vi "Fluke5000.vi"(4 "error in":T13, 7 "Command":T14) -> (0 "error out":T13, 3 "Response":T11)   [LabVIEW 2018]
uses:
  MOKO_LabViewLibrary/MokoLowLevel/MokoLowLovelControl/MLLC_Command.ctl
  MOKO_LabViewLibrary/MokoLowLevel/MokoLowLovelControl/MLLC_Error.ctl
  MOKO_LabViewLibrary/MokoLowLevel/MokoLowLovelControl/MLLC_Mode.ctl
  MOKO_LabViewLibrary/MokoLowLevel/MokoLowLovelControl/MLLC_Response.ctl
  MOKO_LabViewLibrary/MokoLowLevel/MokoLowLovelControl/MLLC_DriverName.ctl
  MOKO_LabViewLibrary/MokoLowLevel/MokoLowLovelControl/MLLC_Request.ctl
  MOKO_LabViewLibrary/MokoLowLevel/MokoLowLovelControl/MLLC_ErrorCode.ctl
  MOKO_LabViewLibrary/MokoLowLevel/MokoLowLovelControl/MLLC_ResponseInit.ctl
  MOKO_LabViewLibrary/MokoLowLevel/MokoLowLovelControl/MLLC_ConnectCluster.ctl
  MOKO_LabViewLibrary/MokoLowLevel/MokoLowLovelControl/MLLC_InterfaceType.ctl
  MOKO_LabViewLibrary/MokoLowLevel/MokoLowLovelControl/MLLC_OpenedSession.ctl
  MOKO_LabViewLibrary/MokoLowLevel/MokoLowLovelControl/MLLC_InterfaceSettings.ctl
  MOKO_LabViewLibrary/MokoLowLevel/MokoLowLovelControl/MLLC_InterfaceKind.ctl
  data/Models.ctl
panel:
  in  "Settings":T6={"Permanent data"={"Connect"={"InterfaceType"=enum."VISA", "OpenedSession"="COM1", "InterfaceSettings"={"Interface"=enum."GPIB", "EOS 4 read"=enum."LF (\\n)", "EOS 4 write"=enum."LF (\\n)", "TMO, ms"=5000, "Sett"=variant(cluster{"Baud Rate":u32, "Data Bits":u16, "Parity":u16, "Stop Bits":u16, "Flow Control":u16, "Eho":bool} {"Baud Rate"=75, "Data Bits"=0, "Parity"=0, "Stop Bits"=0, "Flow Control"=0, "Eho"=FALSE})}}, "Conn"=2, "Model"=0.0, "Channel"="CH1", "Impedance"="Z1M", "SwitchOFF"=TRUE, "Out"="NORMAL", "OutSignalAuto"=TRUE, "PQ"=FALSE}, "Saved Data"=variant} {"Permanent data"."Conn" items=["2-Wire", "4-Wire", "NONE"]}
  in  "Response Init Array":T7[](array[typedef])=["5500", "5502", "5520", "5522", "5700", "5720", "5730"]
  in  "Error Code":T8=5470
  in  "Request":T9="*idn?"
  in  "Driver Name":T10="Fluke5000"
  in  "Mode":T12=enum."Check"
  # "F5000"
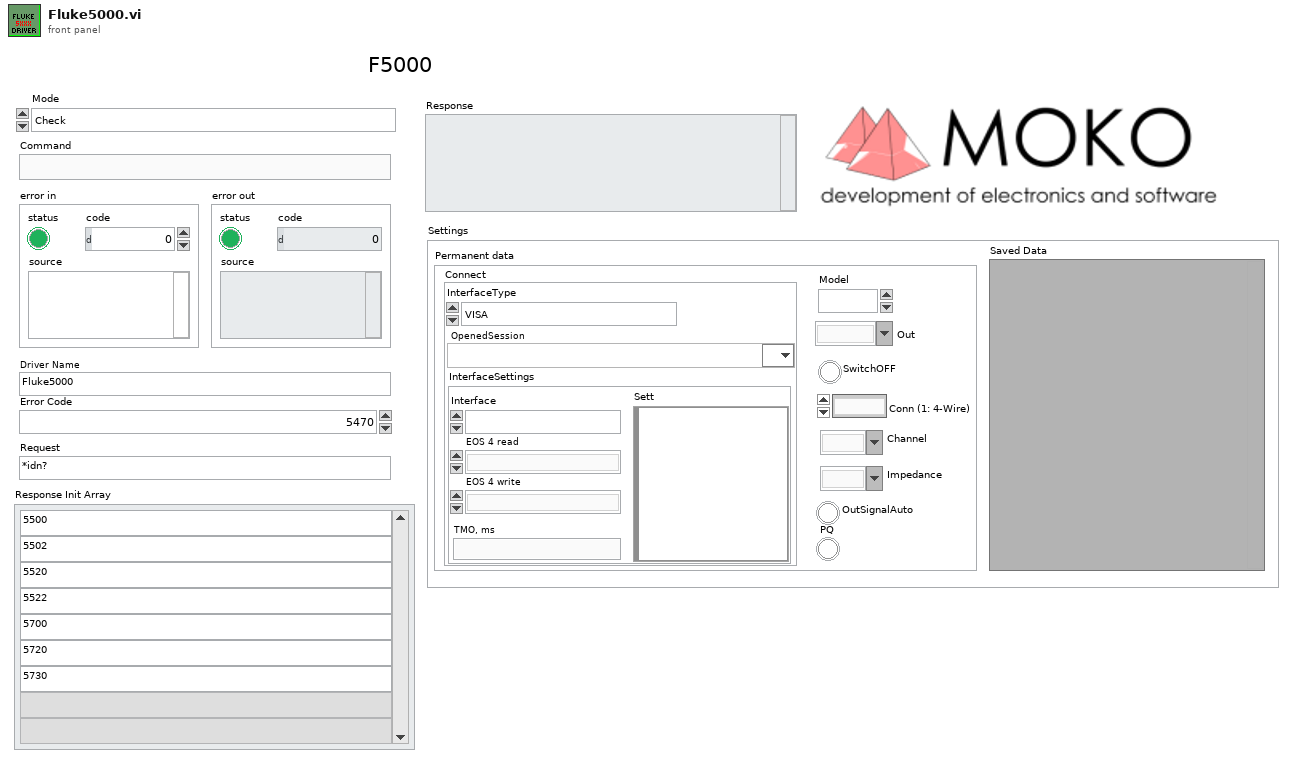
[diagram p1: front panel]
types:
  T1 = typedef "MLLC_ConnectCluster.ctl" = cluster{"InterfaceType":T2, "OpenedSession":T3, "InterfaceSettings":T4}
  T2 = typedef "MLLC_InterfaceType.ctl" = enum16{"VISA", "Prologix USB-GPIB"}
  T3 = typedef "MLLC_OpenedSession.ctl" = refnum<visa-resource-name>
  T4 = typedef "MLLC_InterfaceSettings.ctl" = cluster{"Interface":T5, "EOS 4 read":enum16{"Default (=EOS 4 write)", "CR (\\r)", "LF (\\n)", "None"}, "EOS 4 write":enum16{"CR+LF (\\r\\n)", "CR (\\r)", "LF (\\n)", "None"}, "TMO, ms":i32, "Sett":variant}
  T5 = typedef "MLLC_InterfaceKind.ctl" = enum16{"RS232", "GPIB", "USB", "Ethernet", "another"}
  T6 = cluster{"Permanent data":cluster{"Connect":T1, "Conn":u16, "Model":dbl, "Channel":string, "Impedance":string, "SwitchOFF":bool, "Out":string, "OutSignalAuto":bool, "PQ":bool}, "Saved Data":variant}
  T7 = typedef "MLLC_ResponseInit.ctl" = string
  T8 = typedef "MLLC_ErrorCode.ctl" = u32
  T9 = typedef "MLLC_Request.ctl" = string
  T10 = typedef "MLLC_DriverName.ctl" = string
  T11 = typedef "MLLC_Response.ctl" = string
  T12 = typedef "MLLC_Mode.ctl" = enum16{"get", "set", "close", "Init", "Check"}
  T13 = typedef "MLLC_Error.ctl" = errorcluster
  T14 = typedef "MLLC_Command.ctl" = string
  T15 = enum16{"CR+LF (\\r\\n)", "CR (\\r)", "LF (\\n)", "None"}
  T16 = enum16{"Default (=EOS 4 write)", "CR (\\r)", "LF (\\n)", "None"}
  T17 = cluster{"Connect":T1, "Conn":u16, "Model":dbl, "Channel":string, "Impedance":string, "SwitchOFF":bool, "Out":string, "OutSignalAuto":bool, "PQ":bool}
  T18 = typedef "Models.ctl" = enum16{"5500", "5520", "5700", "5720", "5502", "5522", "5730"}
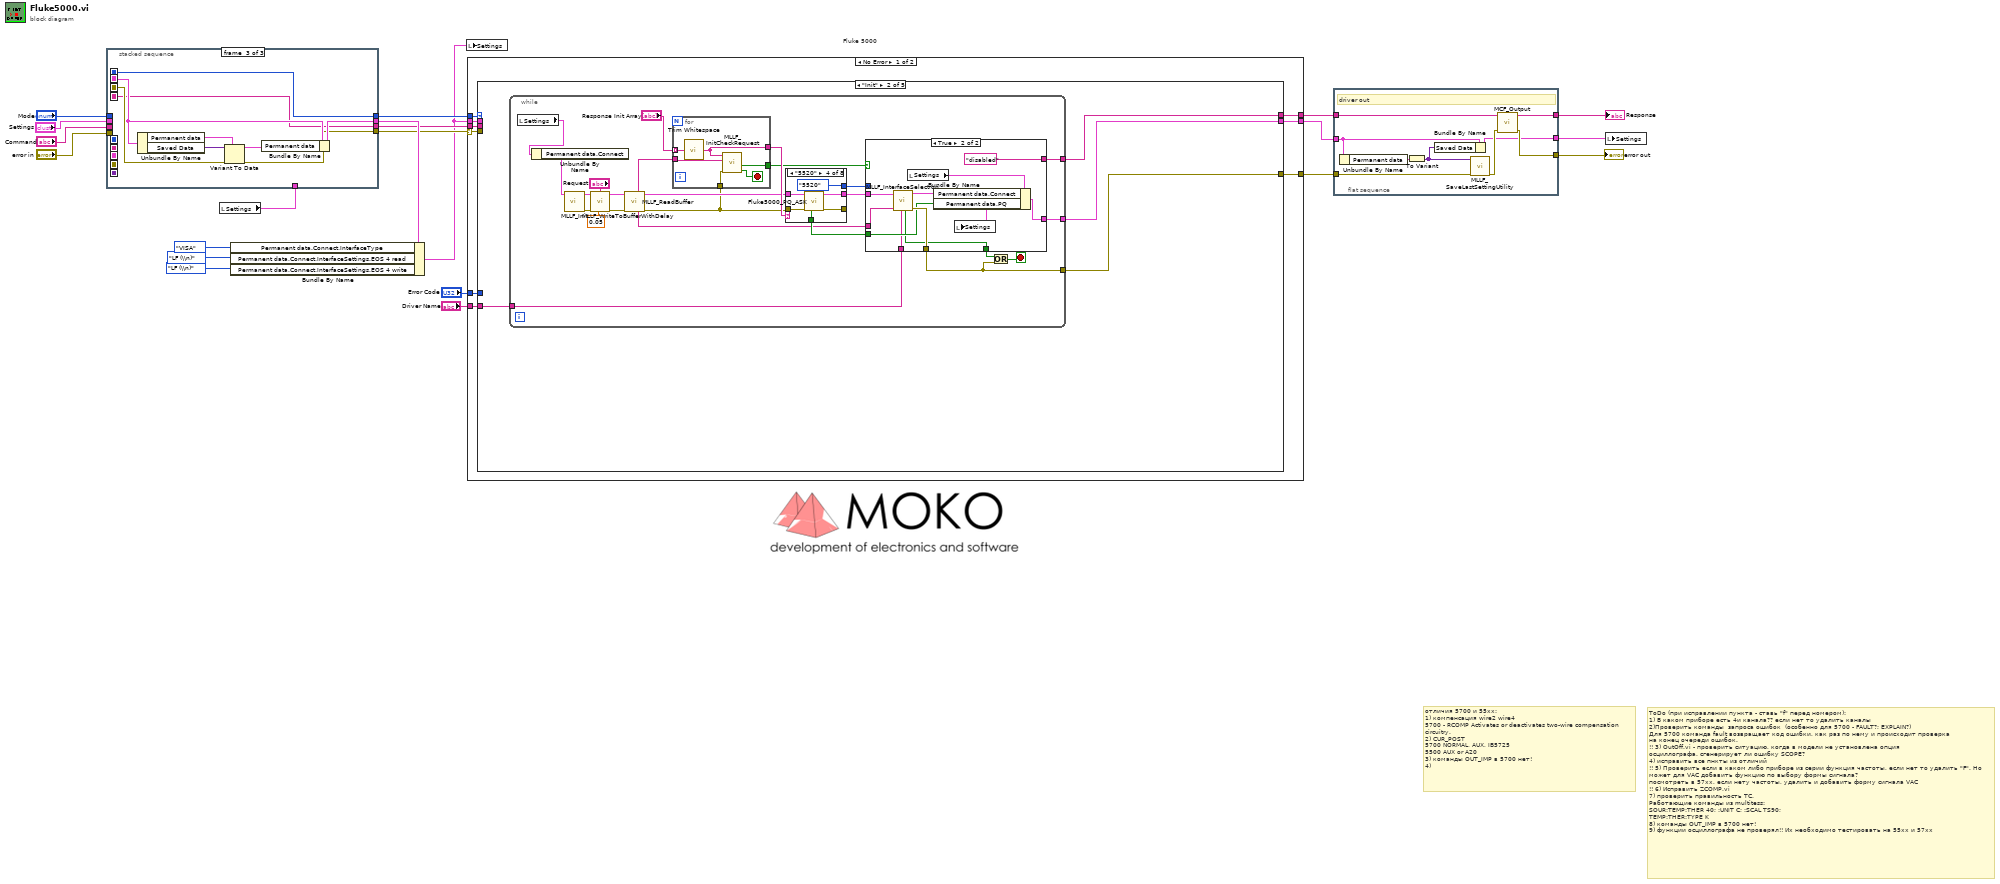
[diagram p0: block diagram]
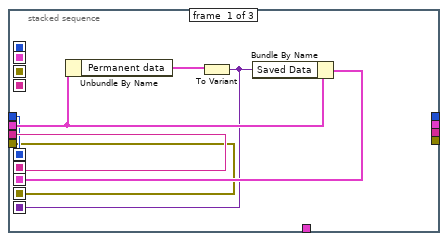
[diagram p2: hidden frame]
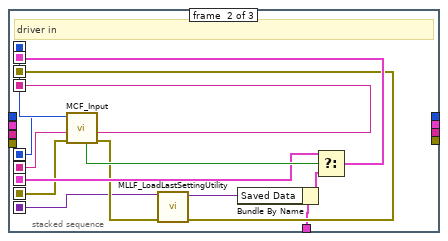
[diagram p3: hidden frame]
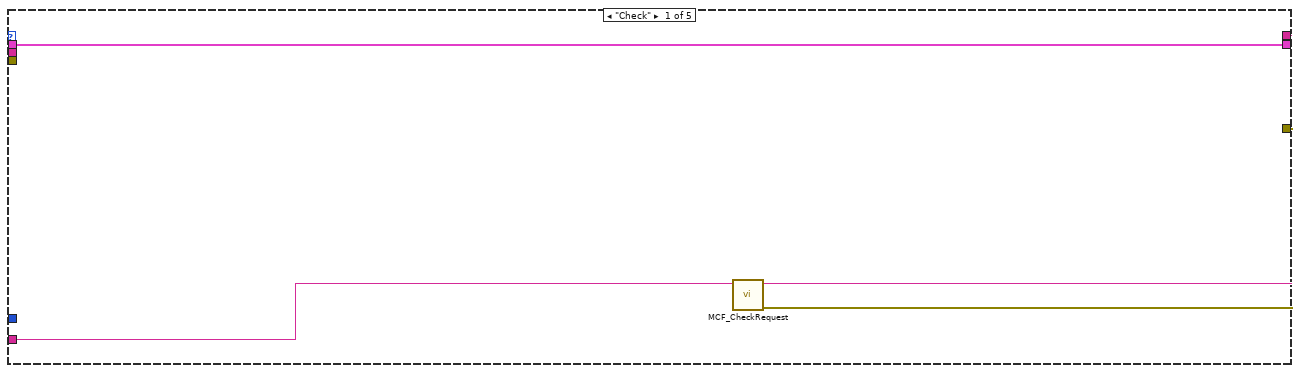
[diagram p4: hidden frame]
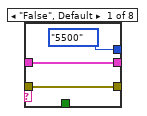
[diagram p5: hidden frame]
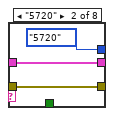
[diagram p6: hidden frame]
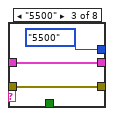
[diagram p7: hidden frame]
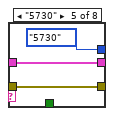
[diagram p8: hidden frame]
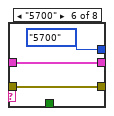
[diagram p9: hidden frame]
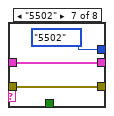
[diagram p10: hidden frame]
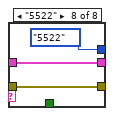
[diagram p11: hidden frame]
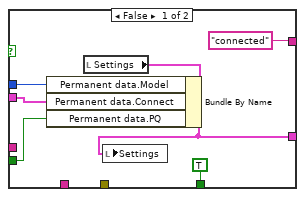
[diagram p12: hidden frame]
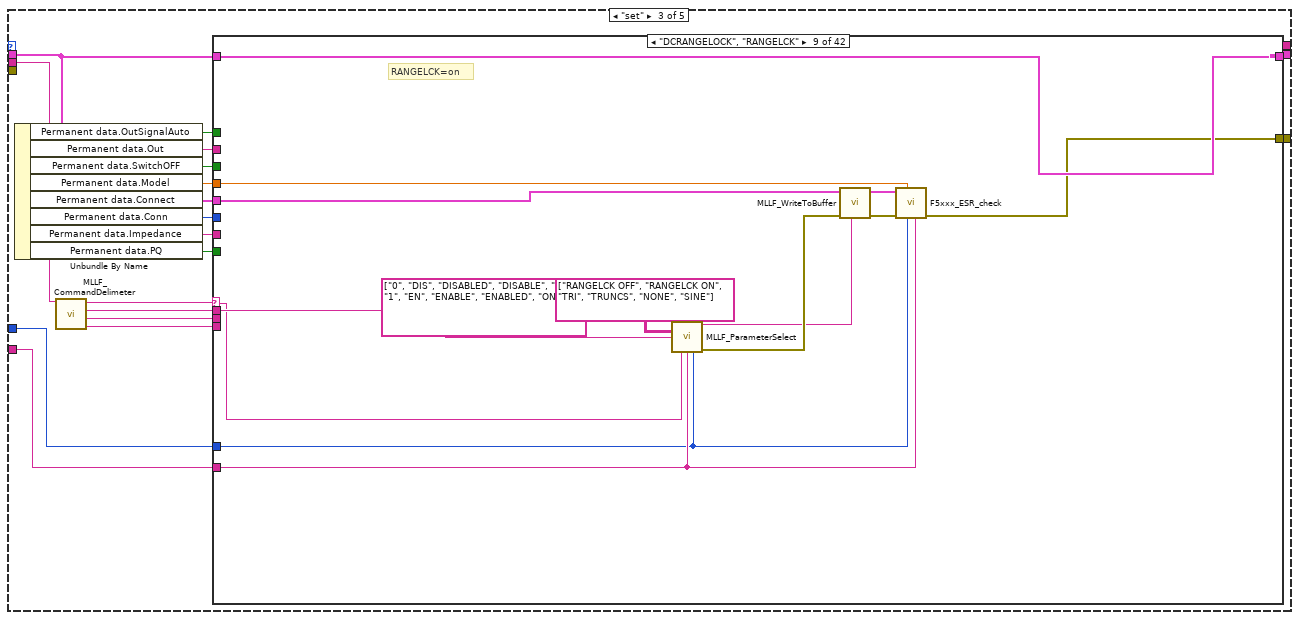
[diagram p13: hidden frame]
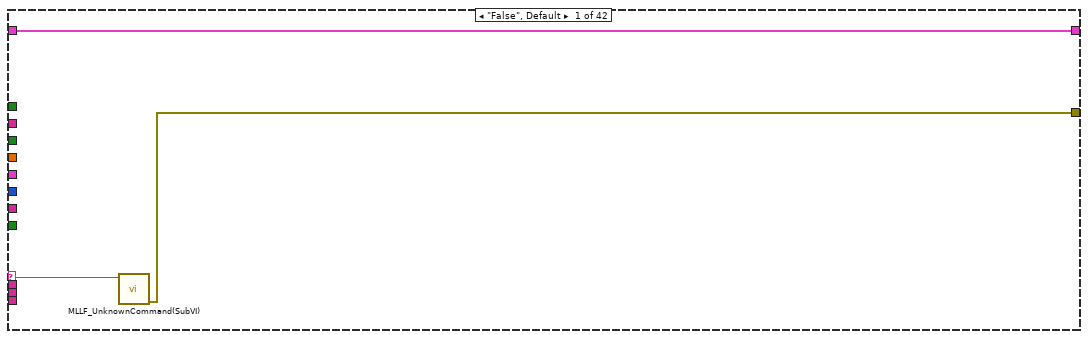
[diagram p14: hidden frame]
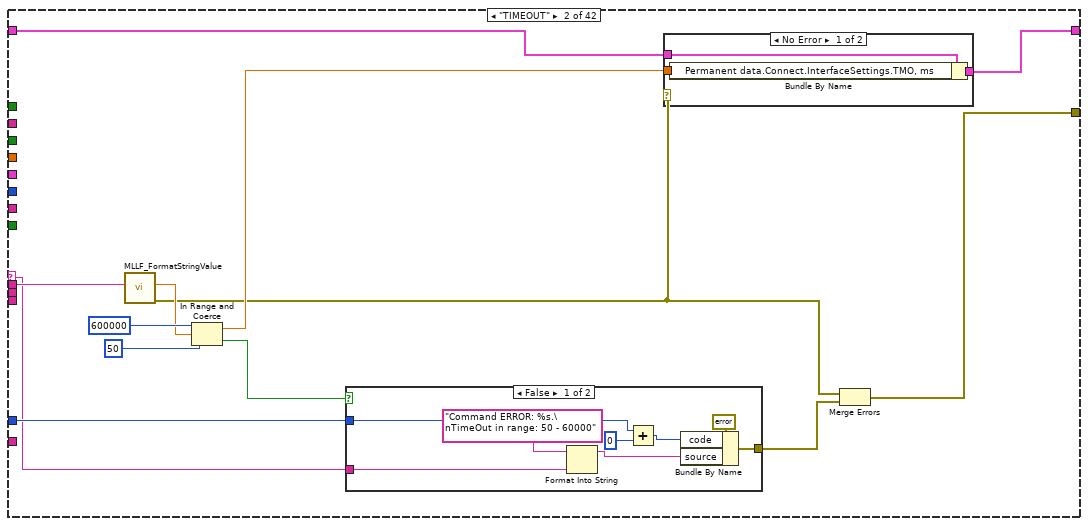
[diagram p15: hidden frame]
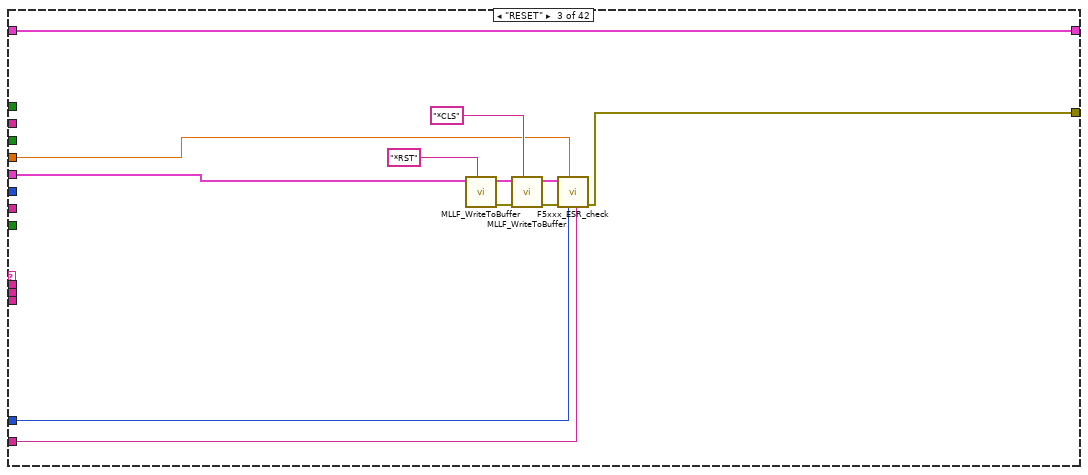
[diagram p18: hidden frame]
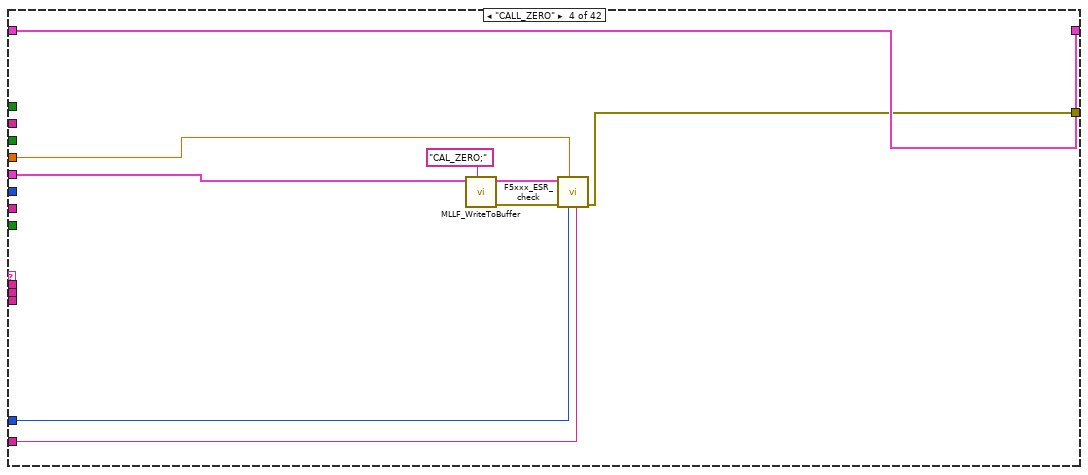
[diagram p19: hidden frame]
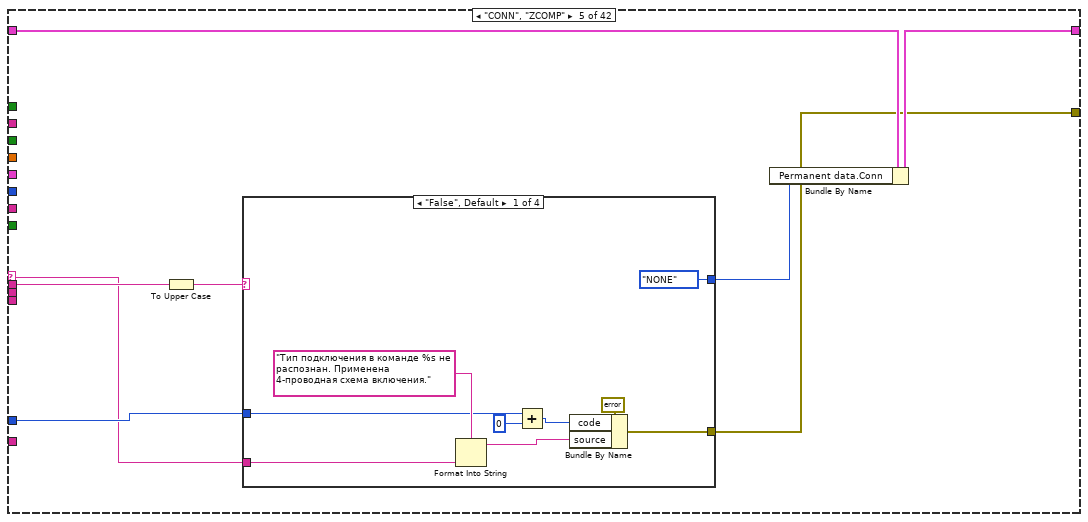
[diagram p20: hidden frame]
diagram:
  # "ToDo (при исправлении пункта - ставь \"f\" перед номером):\n1) В каком приборе есть 4и канала?? если нет то удалить каналы\n2)Проверить команды  запроса ошибок  (особенно для 5700 - FAULT?; EXPLAIN?)\nДля 5700 команда fault возвращает код ошибки, как раз по нему и происходит проверка \nна конец очереди ошибок.\n!! 3) OutOff.vi - проверить ситуацию, когда в модели не установлена опция \nосциллографа. сгенерирует ли ошибку SCOPE?\n4) исправить все пнкты из отличий\n!! 5) Проверить если в каком либо приборе из серии функция частоты, если нет то удалить \"F\". Но \nможет для VAC добавить функцию по выбору формы сигнала?\nпосмотреть в 57хх, если нету частоты, удалить и добавить форму сигнала VAC \n!! 6) Исправить ZCOMP.vi\n7) проверить правильность TC.\nРаботающие команды из multitess: \nSOUR:TEMP:THER 40; :UNIT C; :SCAL TS90;\nTEMP:THER:TYPE K\n8) команды OUT_IMP в 5700 нет! \n9) функции осциллографа не проверял!! Их необходимо тестировать на 55xx и 57xx"
  # "отличия 5700 и 55xx:\n1) компенсация wire2 wire4 \n5700 - RCOMP Activates or deactivates two-wire compensation\ncircuitry.\n2) CUR_POST \n5700 NORMAL, AUX, IB5725\n5500 AUX or A20\n3) команды OUT_IMP в 5700 нет! \n4)"
  # "Fluke 5000"
  n1 = local read "Settings"() -> (w3:T6)
  n2 = stacked-sequence {
    seq-local: [w24 _ _] -> [_ w40 _]
    seq-local: [w23 _ _] -> [_ w41 _]
    seq-local: [w26 _ _] -> [_ w36 _]
    seq-local: [w22 _ _] -> [_ w35 _]
    seq-local: [w25 _ _] -> [_ w30 _]
    seq-local: [_ w31 _] -> [_ _ w47]
    seq-local: [_ w42 _] -> [_ _ w44]
    seq-local: [_ w39 _] -> [_ _ w43]
    seq-local: [_ w38 _] -> [_ _ w48]
    tunnel: "Command" -> [w24 _ _]
    tunnel: "Mode" -> [w23 _ _]
    tunnel: "error in" -> [w22 _ _]
    tunnel: "Settings" -> [w27 _ _]
    tunnel: w3 -> [_ w29 _]
    tunnel: [_ _ w43] -> w11
    tunnel: [_ _ w46] -> w12
    tunnel: [_ _ w45] -> w10
    tunnel: [_ _ w44] -> w13
    frame #0 {
      n3 = Unbundle By Name(w27) -> ("Permanent data"=w28:T17)
      n4 = To Variant(anything=w28) -> (Variant=w25:variant)
      n5 = Bundle By Name(cluster=w27, "Saved Data"=w25) -> (w26:T6)
    }
    frame #1 {
      # "driver in"
      n6 = call "MCF_Input.vi"("Error In"=w35, "Command in"=w40, "Mode in"=w41) -> ("Error Out"=w34:errorcluster, "Command out"=w39:string, "Mode out"=w42:T12, "Boolean"=w37:bool)  [unwired: 5 in]
      n7 = call "MLLF_LoadLastSettingUtility.vi"("Error In"=w34, "Save data in"=w30) -> ("Error Out"=w31:errorcluster, "Save data out"=w33:variant)  [unwired: 8 in]
      n8 = Bundle By Name(cluster=w29, "Saved Data"=w33) -> (w32:T6)
      n9 = Select(t=w36, s=w37, f=w32) -> (s? t:f=w38:T6)
    }
    frame #2 {
      n10 = Unbundle By Name(w48) -> ("Permanent data"=w49:T17, "Saved Data"=w51:variant)
      n11 = Variant To Data(error in=w47, type=w49, Variant=w51) -> (data=w50:T17, error out=w45:errorcluster)
      n12 = Bundle By Name(cluster=w48, "Permanent data"=w50) -> (w46:T6)
    }
  }
  n13 = Bundle By Name(cluster=w12, "Permanent data.Connect.InterfaceType"=MLLC_InterfaceType."VISA" ("Connect.InterfaceType"), "Permanent data.Connect.InterfaceSettings.EOS 4 read"=T16."LF (\\n)" ("Connect.InterfaceSettings.EOS 4 read"), "Permanent data.Connect.InterfaceSettings.EOS 4 write"=T15."LF (\\n)" ("Connect.InterfaceSettings.EOS 4 write")) -> (w2:T6)
  n14 = local write "Settings"(w2) -> ()
  n15 = case shown="No Error" w10 {
    selector: w10 -> [w58 w1639]
    tunnel: w13 -> [w60 _]
    tunnel: w11 -> [w59 _]
    tunnel: w2 -> [w55 w1638]
    tunnel: "Error Code" -> [w57 _]
    tunnel: "Driver Name" -> [w56 _]
    tunnel: [w54 _] -> w9
    tunnel: [w53 w1638] -> w8
    tunnel: [w52 w1639] -> w7
    frame No Error {
      n16 = case shown="\"Init\"" w60 {
        tunnel: [w62 w66 _ w1522 _] -> w54
        tunnel: [w63 w68 w145 w1521 w1636] -> w52
        tunnel: w59 -> [_ _ w159 w1530 _]
        tunnel: w58 -> [_ _ _ _ _]
        tunnel: w57 -> [_ _ w158 w1527 w1634]
        tunnel: w56 -> [w61 w65 w155 w1526 w1633]
        tunnel: w55 -> [w64 _ w157 w1529 w1635]
        tunnel: [w64 w67 w156 w1528 w1635] -> w53
        frame "Check" {
          n17 = call "MCF_CheckRequest.vi"("Driver Name"=w61) -> ("Error Out"=w63:errorcluster, "Output String"=w62:string)  [unwired: 9 in]
        }
        frame "Init" {
          n18 = while {
            tunnel: [w83] -> w68
            tunnel: [w75] -> w67
            tunnel: [w74] -> w66
            tunnel: w65 -> [w70]
            stop <- w84 stop-if-true
            n19 = local read "Settings"() -> (w71:T6)
            n20 = Unbundle By Name(w71) -> ("Permanent data.Connect"=w76:T1)
            n21 = call "MLLF_Init.vi"("DriverConnect in"=w76) -> ("Error Out"=w87:errorcluster, "DriverConnect out"=w86:T1)  [unwired: 7 in]
            n22 = call "MLLF_WriteToBufferWithDelay.vi"("Delay Time ( 0,05 s)"=0.05 ("Delay Time (s)"), "Command"="Request", "Error In"=w87, "DriverConnect in"=w86) -> ("Error Out"=w90:errorcluster, "DriverConnect out"=w89:T1)  [unwired: 6 in]
            n23 = call "MLLF_ReadBuffer.vi"("Error In"=w90, "DriverConnect in"=w89) -> ("Error Out"=w73:errorcluster, "DriverConnect out"=w79:T1, "String"=w69:string)  [unwired: 6 in]
            n24 = for {
              tunnel: "Response Init Array" -> [w96] mode=indexing
              tunnel: [w95] -> w88
              tunnel: w69 -> [w97]
              tunnel: w73 -> [w94]
              tunnel: [w93] -> w72
              stop <- w92 stop-if-true
              n25 = call <vilib>:"Trim Whitespace.vi"("string"=w96) -> ("trimmed string"=w95:string)  [unwired: 1 in]
              n26 = call "MLLF_InitCheckRequest.vi"("error in (no error)"=w94, "Answer"=w97, "Response Init"=w95) -> ("Design ARRAY STOP?"=w92:bool, "Design Interf ARRAY?"=w93:bool)  [unwired: 5 in, 2 out]
            }
            n27 = case shown="\"5520\"" w88 {
              tunnel: [Models."5500" ("Model") Models."5720" ("Model") Models."5500" ("Model") Models."5520" ("Model") Models."5730" ("Model") Models."5700" ("Model") Models."5502" ("Model") Models."5522" ("Model")] -> w85
              tunnel: [_ _ _ w111 _ _ _ _] -> w80
              tunnel: w79 -> [w99 w102 w105 w110 w114 w117 w120 w123]
              tunnel: w73 -> [w98 w101 w104 w109 w113 w116 w119 w122]
              tunnel: [w98 w101 w104 w108 w113 w116 w119 w122] -> _
              tunnel: [w99 w102 w105 w107 w114 w117 w120 w123] -> w78
              frame "False", Default {
              }
              frame "5720" {
              }
              frame "5500" {
              }
              frame "5520" {
                n28 = call "Fluke5000_PQ_ASK.vi"("Error In"=w109, "DriverConnect in"=w110) -> ("Error Out"=w108:errorcluster, "DriverConnect out"=w107:T1, "Boolean"=w111:bool)  [unwired: 7 in]
              }
              frame "5730" {
              }
              frame "5700" {
              }
              frame "5502" {
              }
              frame "5522" {
              }
            }
            n29 = case shown="True" w72 {
              tunnel: w78 -> [w128 w141]
              tunnel: [_ w139] -> w83
              tunnel: w85 -> [w129 _]
              tunnel: [TRUE w136] -> w82
              tunnel: w80 -> [w127 w138]
              tunnel: [w125 w135] -> w75
              tunnel: ["connected" "disabled"] -> w74
              tunnel: w70 -> [_ w133]
              tunnel: w69 -> [_ w132]
              frame False {
                n30 = local read "Settings"() -> (w126:T6)
                n31 = Bundle By Name(cluster=w126, "Permanent data.Model"=w129, "Permanent data.Connect"=w128, "Permanent data.PQ"=w127) -> (w125:T6)
                n32 = local write "Settings"(w125) -> ()
              }
              frame True {
                n33 = call "MLLF_InterfaceSelection.vi"("Driver Name"=w133, "Answer:"=w132, "DriverConnect in"=w141) -> ("error out"=w139:T13, "DriverConnect out"=w140:T1, "stop init?"=w136:bool)  [unwired: 4 in, 2 out]
                n34 = local read "Settings"() -> (w134:T6)
                n35 = Bundle By Name(cluster=w134, "Permanent data.Connect"=w140, "Permanent data.PQ"=w138) -> (w135:T6)
                n36 = local write "Settings"(w135) -> ()
              }
            }
            n37 = Or(x=w82, y=w83) -> (x .or. y?=w84:bool)
          }
        }
        frame "set" {
          n38 = Unbundle By Name(w157) -> ("Permanent data.OutSignalAuto"=w148:bool, "Permanent data.Out"=w149:string, "Permanent data.SwitchOFF"=w150:bool, "Permanent data.Model"=w151:dbl, "Permanent data.Connect"=w154:T1, "Permanent data.Conn"=w153:u16, "Permanent data.Impedance"=w152:string, "Permanent data.PQ"=w147:bool)
          n39 = call "MLLF_CommandDelimeter.vi"("command with param"=w159) -> ("param 3"=w143:string, "param 2"=w144:string, "param 1"=w142:string, "command"=w146:string)  [unwired: 6 in, 1 out]
          n40 = case shown="\"DCRANGELOCK\", \"RANGELCK\"" w146 {
            selector: w146 -> [w161 w163 _ _ w209 w229 _ _ w259 w273 w287 w301 w315 w329 w343 w359 w375 _ _ w449 _ _ _ _ w851 w1015 w1034 w1071 w1106 _ w1166 w1192 _ _ _ _ _ _ _ _ _ _]
            tunnel: w142 -> [_ w166 _ _ w213 w234 _ _ w263 w278 w291 w305 w319 w333 w348 w364 w377 _ w393 w454 w718 w752 w775 w813 w850 w1014 w1042 w1064 w1099 w1134 w1158 w1196 w1220 _ w1249 w1281 w1303 w1339 w1377 _ w1418 w1474]
            tunnel: [w160 w169 w190 w204 w211 w231 w250 w257 w265 w274 w293 w307 w321 w335 w344 w360 w381 _ w391 w457 w734 w753 w793 w811 w844 w999 w1046 w1081 w1116 w1135 w1176 w1195 w1222 _ w1253 w1285 w1321 w1357 w1389 _ w1424 w1480] -> w145
            tunnel: w158 -> [_ w170 w192 w206 w214 w232 w248 w255 w268 w282 w296 w310 w324 w338 w350 w366 w382 _ w395 w456 w731 w759 w790 w815 w853 w1017 w1044 w1074 w1109 w1139 w1162 w1198 w1224 _ w1252 w1284 w1320 w1356 w1388 _ w1416 w1472]
            tunnel: w157 -> [w162 w174 w199 w208 w215 w240 w251 w258 w272 w286 w300 w314 w328 w342 w346 w362 w380 w390 w409 w460 w738 w762 w797 w829 w856 w1020 w1045 w1080 w1115 w1141 w1175 w1204 w1226 w1237 w1257 w1289 w1325 w1361 w1393 w1406 w1427 w1483]
            tunnel: [w162 w175 w199 w208 w216 w241 w251 w258 w272 w286 w300 w314 w328 w342 w345 w361 w379 w390 w409 w460 w738 w762 w797 w829 w856 w1020 w1045 w1080 w1115 w1141 w1175 w1204 w1226 w1237 w1257 w1289 w1325 w1361 w1393 w1406 w1427 w1483] -> w156
            tunnel: w154 -> [_ _ w188 w202 _ _ w247 w254 w260 w275 w288 w302 w316 w330 _ _ _ _ w410 w452 w739 w755 w798 w831 w848 w1021 w1053 w1087 w1122 w1137 w1181 w1193 w1218 _ w1259 w1291 w1327 w1363 w1395 _ w1410 w1466]
            tunnel: w155 -> [_ _ w191 w205 _ w233 w249 w256 w269 w283 w297 w311 w325 w339 w351 w367 w383 _ w394 w455 w732 w760 w791 w814 w852 w1016 w1043 w1075 w1110 w1140 w1170 w1199 w1225 _ w1251 w1283 w1319 w1355 w1387 _ w1415 w1471]
            tunnel: w153 -> [_ _ _ _ _ _ _ _ _ _ _ _ _ _ _ _ _ _ _ _ _ _ _ _ _ w1019 w1037 w1072 w1107 _ w1167 _ _ _ _ _ _ _ _ _ _ _]
            tunnel: w152 -> [_ _ _ _ _ _ _ _ _ _ _ _ _ _ _ _ _ _ _ _ _ _ _ _ _ _ _ _ _ _ _ _ _ _ w1243 w1275 w1313 w1349 w1384 _ _ _]
            tunnel: w151 -> [_ _ w189 w203 _ _ w246 w253 w271 w285 w299 w313 w327 w341 _ _ _ _ w403 w451 w720 w757 w781 w820 w847 w1012 w1036 w1070 w1105 w1138 w1165 w1197 w1223 _ w1240 w1272 w1307 w1343 w1380 _ w1425 w1481]
            tunnel: w150 -> [_ _ _ _ _ _ _ _ _ _ _ _ _ _ _ _ _ _ w402 w459 w730 _ w789 w818 w855 w1018 w1033 w1068 w1103 _ w1163 _ _ _ w1239 w1271 w1305 w1341 w1375 _ _ _]
            tunnel: w149 -> [_ _ _ _ _ _ _ _ _ _ _ _ _ _ _ _ _ _ w401 w458 _ _ _ w816 w854 _ _ _ _ _ _ _ _ _ _ _ _ _ _ _ _ _]
            tunnel: w148 -> [_ _ _ _ _ _ _ _ _ _ _ _ _ _ _ _ _ _ w392 w453 w719 _ w776 w812 w849 w1013 w1032 w1065 w1100 _ w1159 _ _ _ w1238 w1270 w1304 w1340 w1374 _ _ _]
            tunnel: w147 -> [_ _ _ _ _ _ _ _ _ _ _ _ _ _ _ _ _ _ _ w450 _ _ _ _ w846 _ _ _ _ _ _ _ _ _ _ _ _ _ _ _ _ _]
            tunnel: w144 -> [_ _ _ _ _ _ _ _ _ _ _ _ _ _ _ _ _ _ _ w448 w717 _ w774 _ w845 _ _ w1063 w1098 _ _ _ _ _ _ _ w1302 w1338 _ _ _ _]
            tunnel: w143 -> [_ _ _ _ _ _ _ _ _ _ _ _ _ _ _ _ _ _ _ w447 _ _ w773 _ _ _ _ _ _ _ _ _ _ _ _ _ _ _ _ _ _ _]
            frame "False", Default {
              n41 = call "MLLF_UnknownCommand(SubVI).vi"("Unknown command"=w161) -> ("error out"=w160:errorcluster)  [unwired: 10 in]
            }
            frame "TIMEOUT" {
              n42 = call "MLLF_FormatStringValue.vi"("String Value"=w166) -> ("error out"=w164:T13, "number"=w165:dbl)  [unwired: 8 in, 1 out]
              n43 = In Range and Coerce(upper limit=600000, x=w165, lower limit=50) -> (coerced(x)=w171:dbl, In Range?=w167:bool)
              n44 = case shown="False" w167 {
                tunnel: [w182 _] -> w168
                tunnel: w170 -> [w181 _]
                tunnel: w163 -> [w180 _]
                frame False {
                  n45 = Format Into String(format string="Command ERROR: %s.\nTimeOut in range: 50 - 60000", w180) -> (resulting string=w184:string)  [unwired: 2 in, 1 out]
                  n46 = Add(x=w181, y=0) -> (x+y=w185:T8)
                  n47 = Bundle By Name(cluster=errorcluster {"status"=TRUE, "code"=0, "source"=""} ("error out"), "code"=w185, "source"=w184) -> (w182:errorcluster)
                }
                frame True {
                }
              }
              n48 = case shown="No Error" w164 {
                tunnel: [w178 w179] -> w175
                tunnel: w174 -> [w177 w179]
                tunnel: w171 -> [w176 _]
                frame No Error {
                  n49 = Bundle By Name(cluster=w177, "Permanent data.Connect.InterfaceSettings.TMO, ms"=w176) -> (w178:T6)
                }
                frame Error {
                }
              }
              n50 = Merge Errors(w164, w168) -> (w169:errorcluster)
            }
            frame "RESET" {
              n51 = call "MLLF_WriteToBuffer.vi"("String"="*RST", "DriverConnect in"=w188) -> ("error out"=w197:T13, "DriverConnect out"=w198:T1)  [unwired: 6 in]
              n52 = call "MLLF_WriteToBuffer.vi"("String"="*CLS" ("write buffer"), "error in"=w197, "DriverConnect in"=w198) -> ("error out"=w194:T13, "DriverConnect out"=w193:T1)  [unwired: 5 in]
              n53 = call "F5xxx_ESR_check.vi"("Driver Name"=w191, "Error Code"=w192, "Model"=w189, "error in"=w194, "DriverConnect in"=w193) -> ("error out"=w190:T13)  [unwired: 5 in, 1 out]
            }
            frame "CALL_ZERO" {
              n54 = call "MLLF_WriteToBuffer.vi"("String"="CAL_ZERO;", "DriverConnect in"=w202) -> ("error out"=w200:T13, "DriverConnect out"=w201:T1)  [unwired: 6 in]
              n55 = call "F5xxx_ESR_check.vi"("Driver Name"=w205, "Error Code"=w206, "Model"=w203, "error in"=w200, "DriverConnect in"=w201) -> ("error out"=w204:T13)  [unwired: 5 in, 1 out]
            }
            frame "CONN", "ZCOMP" {
              n56 = To Upper Case(1:w213) -> (0:w212:string)
              n57 = case shown="\"False\", Default" w212 {
                tunnel: w209 -> [w220 _ _ _]
                tunnel: [w219 _ _ _] -> w211
                tunnel: w214 -> [w218 _ _ _]
                tunnel: [enum16{"2-Wire", "4-Wire", "NONE"}."NONE" ("Conn") enum16{"2-Wire", "4-Wire", "NONE"}."4-Wire" ("Conn") enum16{"2-Wire", "4-Wire", "NONE"}."2-Wire" ("Conn") enum16{"2-Wire", "4-Wire", "NONE"}."NONE" ("Conn")] -> w210
                frame "False", Default {
                  n58 = Format Into String(format string="Тип подключения в команде %s не распознан. Применена 4-проводная схема включения.", w220) -> (resulting string=w222:string)  [unwired: 2 in, 1 out]
                  n59 = Add(x=w218, y=0) -> (x+y=w223:T8)
                  n60 = Bundle By Name(cluster=errorcluster {"status"=TRUE, "code"=0, "source"=""} ("error out"), "code"=w223, "source"=w222) -> (w219:errorcluster)
                }
                frame "4W" {
                }
                frame "2W" {
                }
                frame "NO", "NONE" {
                }
              }
              n61 = Bundle By Name(cluster=w215, "Permanent data.Conn"=w210) -> (w216:T6)
            }
            frame "OUTIMP" {
              # "OutImp=1M"
              n62 = call "MLLF_FormatStringValue.vi"("String Value"=w234, "Format"="%#f" ("format")) -> ("error out"=w236:T13, "String Value Formated"=w237:T14)  [unwired: 7 in, 1 out]
              n63 = call "MLLF_ParameterSelect.vi"("Command to equipment"=string[] ["Z50", "Z1M"] ("Parameters"), "Names"=string[][] [["50"], ["1000000"]], "Input"=w237, "Error In"=w236, "Command"=w229, "Driver Name"=w233, "Error Code"=w232) -> ("Choice"=w230:string, "Error Out"=w231:errorcluster)  [unwired: 7 in]
              n64 = case shown="Error" w231 {
                tunnel: [w244 w245] -> w241
                tunnel: w240 -> [w243 w245]
                tunnel: w230 -> [w242 _]
                frame No Error {
                  n65 = Bundle By Name(cluster=w243, "Permanent data.Impedance"=w242) -> (w244:T6)
                }
                frame Error {
                }
              }
            }
            frame "STOP" {
              n66 = call "Out_Off_F5xxx.vi"("Driver Name"=w249, "Error Code"=w248, "Model"=w246, "DriverConnect in"=w247) -> ("error out"=w250:T13)  [unwired: 6 in, 1 out]
            }
            frame "OPERATE", "RUN" {
              n67 = call "Out_On_F5xxx.vi"("DriverConnect in"=w254, "Model"=w253, "Output Signal Auto ON"=TRUE, "Error Code"=w255, "Driver Name"=w256) -> ("error out"=w257:T13)  [unwired: 9 in, 1 out]
            }
            frame "DCRANGELOCK", "RANGELCK" {
              # "RANGELCK=on"
              n68 = call "MLLF_ParameterSelect.vi"("Command to equipment"=string[] ["RANGELCK OFF", "RANGELCK ON", "TRI", "TRUNCS", "NONE", "SINE"] ("Parameters"), "Names"=string[][] [["0", "DIS", "DISABLED", "DISABLE", "OFF"], ["1", "EN", "ENABLE", "ENABLED", "ON"]], "Input"=w263, "Command"=w259, "Driver Name"=w269, "Error Code"=w268) -> ("Choice"=w261:string, "Error Out"=w262:errorcluster)  [unwired: 8 in]
              n69 = call "MLLF_WriteToBuffer.vi"("String"=w261, "error in"=w262, "DriverConnect in"=w260) -> ("error out"=w267:T13, "DriverConnect out"=w266:T1)  [unwired: 5 in]
              n70 = call "F5xxx_ESR_check.vi"("Driver Name"=w269, "Error Code"=w268, "Model"=w271, "error in"=w267, "DriverConnect in"=w266) -> ("error out"=w265:T13)  [unwired: 5 in, 1 out]
            }
            frame "PQ_EN" {
              # "PQ_EN=OFF"
              n71 = call "MLLF_ParameterSelect.vi"("Command to equipment"=string[] ["PQ OFF", "PQ CH", "PQ DAMPL", "TRUNCS", "NONE", "SINE"] ("Parameters"), "Names"=string[][] [["0", "DIS", "DISABLED", "DISABLE", "OFF"], ["CH", "CH", "CH", "CH", "CH"], ["DAMPL", "DAMPL", "DAMPL", "DAMPL", "DAMPL"]], "Input"=w278, "Command"=w273, "Driver Name"=w283, "Error Code"=w282) -> ("Choice"=w276:string, "Error Out"=w277:errorcluster)  [unwired: 8 in]
              n72 = call "MLLF_WriteToBuffer.vi"("String"=w276, "error in"=w277, "DriverConnect in"=w275) -> ("error out"=w281:T13, "DriverConnect out"=w280:T1)  [unwired: 5 in]
              n73 = call "F5xxx_ESR_check.vi"("Driver Name"=w283, "Error Code"=w282, "Model"=w285, "error in"=w281, "DriverConnect in"=w280) -> ("error out"=w274:T13)  [unwired: 5 in, 1 out]
              n74 = case shown="Error" w274 {
                frame No Error {
                }
                frame Error {
                }
              }
            }
            frame "EXSENSE" {
              # "EXTSENSE=on"
              n75 = call "MLLF_ParameterSelect.vi"("Command to equipment"=string[] ["EXTSENSE OFF", "EXTSENSE ON", "TRI", "TRUNCS", "NONE", "SINE"] ("Parameters"), "Names"=string[][] [["0", "DIS", "DISABLED", "DISABLE", "OFF"], ["1", "EN", "ENABLE", "ENABLED", "ON"]], "Input"=w291, "Command"=w287, "Driver Name"=w297, "Error Code"=w296) -> ("Choice"=w289:string, "Error Out"=w290:errorcluster)  [unwired: 8 in]
              n76 = call "MLLF_WriteToBuffer.vi"("String"=w289, "error in"=w290, "DriverConnect in"=w288) -> ("error out"=w295:T13, "DriverConnect out"=w294:T1)  [unwired: 5 in]
              n77 = call "F5xxx_ESR_check.vi"("Driver Name"=w297, "Error Code"=w296, "Model"=w299, "error in"=w295, "DriverConnect in"=w294) -> ("error out"=w293:T13)  [unwired: 5 in, 1 out]
            }
            frame "LCOMP" {
              # "LCOMP=on"
              n78 = call "MLLF_ParameterSelect.vi"("Command to equipment"=string[] ["LCOMP OFF", "LCOMP ON", "TRI", "TRUNCS", "NONE", "SINE"] ("Parameters"), "Names"=string[][] [["0", "DIS", "DISABLED", "DISABLE", "OFF"], ["1", "EN", "ENABLE", "ENABLED", "ON"]], "Input"=w305, "Command"=w301, "Driver Name"=w311, "Error Code"=w310) -> ("Choice"=w303:string, "Error Out"=w304:errorcluster)  [unwired: 8 in]
              n79 = call "MLLF_WriteToBuffer.vi"("String"=w303, "error in"=w304, "DriverConnect in"=w302) -> ("error out"=w309:T13, "DriverConnect out"=w308:T1)  [unwired: 5 in]
              n80 = call "F5xxx_ESR_check.vi"("Driver Name"=w311, "Error Code"=w310, "Model"=w313, "error in"=w309, "DriverConnect in"=w308) -> ("error out"=w307:T13)  [unwired: 5 in, 1 out]
            }
            frame "RCOMP" {
              # "RCOMP=on"
              n81 = call "MLLF_ParameterSelect.vi"("Command to equipment"=string[] ["RCOMP OFF", "RCOMP ON", "TRI", "TRUNCS", "NONE", "SINE"] ("Parameters"), "Names"=string[][] [["0", "DIS", "DISABLED", "DISABLE", "off"], ["1", "EN", "ENABLED", "ENABLE", "on"]], "Input"=w319, "Command"=w315, "Driver Name"=w325, "Error Code"=w324) -> ("Choice"=w317:string, "Error Out"=w318:errorcluster)  [unwired: 8 in]
              n82 = call "MLLF_WriteToBuffer.vi"("String"=w317, "error in"=w318, "DriverConnect in"=w316) -> ("error out"=w323:T13, "DriverConnect out"=w322:T1)  [unwired: 5 in]
              n83 = call "F5xxx_ESR_check.vi"("Driver Name"=w325, "Error Code"=w324, "Model"=w327, "error in"=w323, "DriverConnect in"=w322) -> ("error out"=w321:T13)  [unwired: 5 in, 1 out]
            }
            frame "EXTSENSE" {
              # "EXTSENSE=on"
              n84 = call "MLLF_ParameterSelect.vi"("Command to equipment"=string[] ["EXTSENSE OFF", "EXTSENSE ON", "TRI", "TRUNCS", "NONE", "SINE"] ("Parameters"), "Names"=string[][] [["0", "DIS", "DISABLED", "DISABLE", "off"], ["1", "EN", "ENABLED", "ENABLE", "on"]], "Input"=w333, "Command"=w329, "Driver Name"=w339, "Error Code"=w338) -> ("Choice"=w331:string, "Error Out"=w332:errorcluster)  [unwired: 8 in]
              n85 = call "MLLF_WriteToBuffer.vi"("String"=w331, "error in"=w332, "DriverConnect in"=w330) -> ("error out"=w337:T13, "DriverConnect out"=w336:T1)  [unwired: 5 in]
              n86 = call "F5xxx_ESR_check.vi"("Driver Name"=w339, "Error Code"=w338, "Model"=w341, "error in"=w337, "DriverConnect in"=w336) -> ("error out"=w335:T13)  [unwired: 5 in, 1 out]
            }
            frame "SwitchOFF", "SwOff" {
              # "SwitchOFF=enable"
              n87 = call "MLLF_ParameterSelect.vi"("Command to equipment"=string[] ["OFF", "ON", "TRI", "TRUNCS", "NONE", "SINE"] ("Parameters"), "Names"=string[][] [["0", "DIS", "DISABLED", "DISABLE", "OFF"], ["1", "EN", "ENABLE", "ENABLED", "ON"]], "Input"=w348, "Command"=w343, "Driver Name"=w351, "Error Code"=w350) -> ("Choice"=w347:string, "Error Out"=w344:errorcluster)  [unwired: 8 in]
              n88 = case shown="No Error" w344 {
                tunnel: w347 -> [w357 _]
                tunnel: w346 -> [w355 w358]
                tunnel: [w354 w358] -> w345
                frame No Error {
                  n89 = Equal?(x="ON", y=w357) -> (x = y?=w353:bool)
                  n90 = Bundle By Name(cluster=w355, "Permanent data.SwitchOFF"=w353) -> (w354:T6)
                }
                frame Error {
                }
              }
            }
            frame "OutSignalAuto" {
              # "OutSignalAuto=OFF"
              n91 = call "MLLF_ParameterSelect.vi"("Command to equipment"=string[] ["OFF", "ON", "TRI", "TRUNCS", "NONE", "SINE"] ("Parameters"), "Names"=string[][] [["0", "DIS", "DISABLED", "DISABLE", "OFF"], ["1", "EN", "ENABLE", "ENABLED", "ON"]], "Input"=w364, "Command"=w359, "Driver Name"=w367, "Error Code"=w366) -> ("Choice"=w363:string, "Error Out"=w360:errorcluster)  [unwired: 8 in]
              n92 = case shown="No Error" w360 {
                tunnel: w363 -> [w373 _]
                tunnel: w362 -> [w371 w374]
                tunnel: [w370 w374] -> w361
                frame No Error {
                  n93 = Equal?(x="ON", y=w373) -> (x = y?=w369:bool)
                  n94 = Bundle By Name(cluster=w371, "Permanent data.OutSignalAuto"=w369) -> (w370:T6)
                }
                frame Error {
                }
              }
            }
            frame "OUT", "OUTPUT" {
              # "out=norm"
              n95 = To Upper Case(1:w377) -> (0:w376:string)
              n96 = call "MLLF_ParameterSelect.vi"("Command to equipment"=string[] ["NORMAL", "AUX", "IB5725", "A20"] ("Parameters"), "Names"=string[][] [["NORM", "NORMAL"], ["AUX", "AUX"], ["IB5725", "IB5725"], ["A20", "А20"]], "Input"=w376, "Command"=w375, "Driver Name"=w383, "Error Code"=w382) -> ("Choice"=w378:string, "Error Out"=w381:errorcluster)  [unwired: 8 in]
              n97 = case shown="No Error" w381 {
                tunnel: w380 -> [w388 w389]
                tunnel: [w387 w389] -> w379
                tunnel: w378 -> [w386 _]
                frame No Error {
                  n98 = Bundle By Name(cluster=w388, "Permanent data.Out"=w386) -> (w387:T6)
                }
                frame Error {
                }
              }
            }
            frame "<----MAIN FUNCTIONS---->" {
            }
            frame "VDC" {
              # "VDC=5"
              # "OUT 45V, 0 HZ; WAVE NONE;"
              n99 = call "Out_Off_F5xxx.vi"("Driver Name"=w394, "SwitchOFF"=w402, "Error Code"=w395, "Model"=w403, "DriverConnect in"=w410) -> ("error out"=w397:T13, "DriverConnect out"=w398:T1)  [unwired: 5 in]
              n100 = case shown="0, Default" w403 {
                tunnel: w401 -> [w418 _]
                tunnel: [w415 "%.;OUT %#e V, 0 HZ;" ("format string")] -> w400
                tunnel: [w414 w435] -> w399
                tunnel: w398 -> [w413 w435]
                tunnel: w397 -> [w412 w434]
                tunnel: [w411 w434] -> w396
                frame 0, Default {
                  n101 = Equal?(x=w418, y="AUX") -> (x = y?=w416:bool)
                  n102 = case shown="True" w416 {
                    tunnel: ["%.;OUT %#e V, 0 HZ; WAVE NONE;" ("format string") w423] -> w415
                    tunnel: [w420 w429] -> w414
                    tunnel: w413 -> [w420 w433]
                    tunnel: w412 -> [w419 w432]
                    tunnel: [w419 w425] -> w411
                    frame False {
                    }
                    frame True {
                      n103 = call "MLLF_WriteToBuffer.vi"("String"="OUT?" ("y"), "error in"=w432, "DriverConnect in"=w433) -> ("error out"=w431:T13, "DriverConnect out"=w430:T1)  [unwired: 5 in]
                      n104 = call "MLLF_ReadBuffer.vi"("Error In"=w431, "DriverConnect in"=w430) -> ("Error Out"=w426:errorcluster, "DriverConnect out"=w429:T1, "String"=w427:string)  [unwired: 6 in]
                      n105 = call "F5000_Find_V.vi"("Error In"=w426, "String in"=w427) -> ("Error Out"=w425:errorcluster, "String out"=w422:string)  [unwired: 8 in]
                      n106 = Concatenate Strings(w422, ", %.;%#e V, 0 HZ; WAVE NONE;" ("format string")) -> (w423:string)
                    }
                  }
                }
                frame 3, 6 {
                }
              }
              n107 = call "MLLF_FormatStringValue.vi"("error in"=w396, "String Value"=w393, "Format"=w400) -> ("error out"=w404:T13, "String Value Formated"=w405:T14)  [unwired: 6 in, 1 out]
              n108 = for {
                N: 2 -> [_]
                tunnel: w399 -> [w446]
                tunnel: w404 -> [w445]
                tunnel: w405 -> [w444]
                tunnel: [w439] -> w407
                tunnel: [w438] -> w406
                tunnel: w395 -> [w443]
                tunnel: w394 -> [w442]
                tunnel: w403 -> [w437]
                stop <- w438 continue-if-true
                n109 = call "MLLF_WriteToBuffer.vi"("String"=w444, "error in"=w445, "DriverConnect in"=w446) -> ("error out"=w441:T13, "DriverConnect out"=w440:T1)  [unwired: 5 in]
                n110 = call "F5xxx_ESR_check.vi"("Driver Name"=w442, "Error Code"=w443, "Model"=w437, "error in"=w441, "DriverConnect in"=w440) -> ("error out"=w438:T13, "DriverConnect out"=w439:T1)  [unwired: 5 in]
              }
              n111 = call "Out_On_F5xxx.vi"("DriverConnect in"=w407, "Model"=w403, "Output Signal Auto ON"=w392, "error in"=w406, "Error Code"=w395, "Driver Name"=w394) -> ("error out"=w391:T13)  [unwired: 8 in, 1 out]
            }
            frame "VAC" {
              n112 = case shown="Default" w451 {
                tunnel: w451 -> [w476 w631 w687]
                tunnel: w449 -> [w475 w630 _]
                tunnel: w459 -> [w474 w629 w686]
                tunnel: w458 -> [w473 w628 w685]
                tunnel: [w472 w600 w662] -> w457
                tunnel: w456 -> [w471 w627 w684]
                tunnel: w455 -> [w470 w626 w683]
                tunnel: w449 -> [w469 _ _]
                tunnel: w454 -> [w468 w603 w664]
                tunnel: w453 -> [w467 w625 w682]
                tunnel: w452 -> [w466 w624 w681]
                tunnel: w450 -> [w463 _ _]
                tunnel: w448 -> [w462 w602 w663]
                tunnel: w447 -> [w461 w601 _]
                frame Default {
                  n113 = case shown="True" w463 {
                    tunnel: w466 -> [w478 w482]
                    tunnel: [w478 w480] -> w465
                    tunnel: ["OFF" ("String") w479] -> w464
                    frame False {
                    }
                    frame True {
                      n114 = call "MLLF_WriteToBuffer.vi"("String"="PQ?", "DriverConnect in"=w482) -> ("error out"=w484:T13, "DriverConnect out"=w483:T1)  [unwired: 6 in]
                      n115 = call "MLLF_ReadBuffer.vi"("Error In"=w484, "DriverConnect in"=w483) -> ("DriverConnect out"=w480:T1, "String"=w479:string)  [unwired: 6 in, 1 out]
                    }
                  }
                  n116 = case shown="\"OFF\", Default" w464 {
                    tunnel: w465 -> [w510 w569]
                    tunnel: w476 -> [w502 w561]
                    tunnel: w475 -> [_ w555]
                    tunnel: w474 -> [w500 w553]
                    tunnel: w473 -> [w498 w551]
                    tunnel: [w485 w538] -> w472
                    tunnel: w471 -> [w491 w544]
                    tunnel: w470 -> [w490 w543]
                    tunnel: w469 -> [_ _]
                    tunnel: w468 -> [w487 w540]
                    tunnel: w467 -> [w489 w542]
                    tunnel: w462 -> [w486 w541]
                    tunnel: w461 -> [_ w539]
                    frame "CH" {
                      # "F"
                      n117 = Equal?(x=w498, y="AUX") -> (x = y?=w495:bool)
                      n118 = call "Out_Off_F5xxx.vi"("Driver Name"=w490, "SwitchOFF"=w500, "Error Code"=w491, "Model"=w502, "DriverConnect in"=w510) -> ("error out"=w493:T13, "DriverConnect out"=w496:T1)  [unwired: 5 in]
                      n119 = case shown="False" w495 {
                        tunnel: [w513 w518] -> w497
                        tunnel: w496 -> [w513 w519]
                        tunnel: ["%.;OUT %#e V," ("format string") w515] -> w494
                        tunnel: w493 -> [w511 w520]
                        tunnel: [w511 w517] -> w492
                        frame False {
                        }
                        frame True {
                          n120 = call "MLLF_WriteToBuffer.vi"("String"="OUT?" ("y"), "error in"=w520, "DriverConnect in"=w519) -> ("error out"=w521:T13, "DriverConnect out"=w522:T1)  [unwired: 5 in]
                          n121 = call "MLLF_ReadBuffer.vi"("Error In"=w521, "DriverConnect in"=w522) -> ("Error Out"=w525:errorcluster, "DriverConnect out"=w518:T1, "String"=w524:string)  [unwired: 6 in]
                          n122 = call "F5000_Find_V.vi"("Error In"=w525, "String in"=w524) -> ("Error Out"=w517:errorcluster, "String out"=w514:string)  [unwired: 8 in]
                          n123 = Concatenate Strings(w514, ", %.;%#e V," ("format string")) -> (w515:string)
                        }
                      }
                      n124 = call "MLLF_FormatStringValue.vi"("error in"=w492, "String Value"=w487, "Format"=w494) -> ("error out"=w488:T13, "String Value Formated"=w504:T14)  [unwired: 6 in, 1 out]
                      n125 = case shown="2, 3" w502 {
                        tunnel: ["%.;%#e HZ;" ("format string") "%.;%#e HZ;" ("format string")] -> w503
                        frame 0, Default {
                        }
                        frame 2, 3 {
                        }
                      }
                      n126 = Concatenate Strings(w504, w503) -> (w501:string)
                      n127 = call "MLLF_FormatStringValue.vi"("error in"=w488, "String Value"=w486, "Format"=w501) -> ("error out"=w506:T13, "String Value Formated"=w505:T14)  [unwired: 6 in, 1 out]
                      n128 = for {
                        N: 3 -> [_]
                        tunnel: w497 -> [w537]
                        tunnel: w506 -> [w536]
                        tunnel: w505 -> [w535]
                        tunnel: [w529] -> w508
                        tunnel: [w530] -> w507
                        tunnel: w491 -> [w532]
                        tunnel: w490 -> [w531]
                        tunnel: w502 -> [w528]
                        stop <- w530 continue-if-true
                        n129 = call "MLLF_WriteToBuffer.vi"("String"=w535, "error in"=w536, "DriverConnect in"=w537) -> ("error out"=w534:T13, "DriverConnect out"=w533:T1)  [unwired: 5 in]
                        n130 = call "F5xxx_ESR_check.vi"("Driver Name"=w531, "Error Code"=w532, "Model"=w528, "error in"=w534, "DriverConnect in"=w533) -> ("error out"=w530:T13, "DriverConnect out"=w529:T1)  [unwired: 5 in]
                      }
                      n131 = call "Out_On_F5xxx.vi"("DriverConnect in"=w508, "Model"=w502, "Output Signal Auto ON"=w489, "error in"=w507, "Error Code"=w491, "Driver Name"=w490) -> ("error out"=w485:T13)  [unwired: 8 in, 1 out]
                    }
                    frame "OFF", Default {
                      # "F"
                      # "U"
                      n132 = Equal?(x=w551, y="AUX") -> (x = y?=w548:bool)
                      n133 = call "Out_Off_F5xxx.vi"("Driver Name"=w543, "SwitchOFF"=w553, "Error Code"=w544, "Model"=w561, "DriverConnect in"=w569) -> ("error out"=w546:T13, "DriverConnect out"=w549:T1)  [unwired: 5 in]
                      n134 = case shown="True" w548 {
                        tunnel: [w572 w577] -> w550
                        tunnel: w549 -> [w572 w578]
                        tunnel: ["%.;OUT %#e V," ("format string") w574] -> w547
                        tunnel: w546 -> [w570 w579]
                        tunnel: [w570 w576] -> w545
                        frame False {
                        }
                        frame True {
                          n135 = call "MLLF_WriteToBufferWithDelay.vi"("Command"="OUT?" ("y"), "Error In"=w579, "DriverConnect in"=w578) -> ("Error Out"=w580:errorcluster, "DriverConnect out"=w581:T1)  [unwired: 7 in]
                          n136 = call "MLLF_ReadBuffer.vi"("Error In"=w580, "DriverConnect in"=w581) -> ("Error Out"=w584:errorcluster, "DriverConnect out"=w577:T1, "String"=w583:string)  [unwired: 6 in]
                          n137 = call "F5000_Find_V.vi"("Error In"=w584, "String in"=w583) -> ("Error Out"=w576:errorcluster, "String out"=w573:string)  [unwired: 8 in]
                          n138 = Concatenate Strings(w573, ", %.;%#e V," ("format string")) -> (w574:string)
                        }
                      }
                      n139 = call "MLLF_FormatStringValue.vi"("error in"=w545, "String Value"=w540, "Format"=w547) -> ("error out"=w557:T13, "String Value Formated"=w563:T14)  [unwired: 6 in, 1 out]
                      n140 = call "MLLF_ParameterSelect.vi"("Command to equipment"=string[] ["SINE", "SQUARE", "TRI", "TRUNCS", "NONE", "SINE"] ("Parameters"), "Names"=string[][] [["SIN", "SINE"], ["SQU", "SQUARE"], ["TRI", "TRIANGLE"], ["TRUNCS", "TRUNCSIN"], ["NONE", "NO"], ["", ""]], "Input"=w539, "Error In"=w557, "Command"=w555, "Driver Name"=w543, "Error Code"=w544) -> ("Choice"=w554:string, "Error Out"=w556:errorcluster)  [unwired: 7 in]
                      n141 = case shown="2, 3" w561 {
                        tunnel: [w585 "%.;%#e HZ;" ("format string")] -> w562
                        tunnel: w554 -> [w586 _]
                        frame 0, Default {
                          n142 = Concatenate Strings("%.;%#e HZ; WAVE " ("format string"), w586, ";" ("format string")) -> (w585:string)
                        }
                        frame 2, 3 {
                        }
                      }
                      n143 = Concatenate Strings(w563, w562) -> (w558:string)
                      n144 = call "MLLF_FormatStringValue.vi"("error in"=w556, "String Value"=w541, "Format"=w558) -> ("error out"=w565:T13, "String Value Formated"=w564:T14)  [unwired: 6 in, 1 out]
                      n145 = for {
                        N: 3 -> [_]
                        tunnel: w550 -> [w599]
                        tunnel: w565 -> [w598]
                        tunnel: w564 -> [w597]
                        tunnel: [w591] -> w567
                        tunnel: [w592] -> w566
                        tunnel: w544 -> [w594]
                        tunnel: w543 -> [w593]
                        tunnel: w561 -> [w590]
                        stop <- w592 continue-if-true
                        n146 = call "MLLF_WriteToBuffer.vi"("String"=w597, "error in"=w598, "DriverConnect in"=w599) -> ("error out"=w596:T13, "DriverConnect out"=w595:T1)  [unwired: 5 in]
                        n147 = call "F5xxx_ESR_check.vi"("Driver Name"=w593, "Error Code"=w594, "Model"=w590, "error in"=w596, "DriverConnect in"=w595) -> ("error out"=w592:T13, "DriverConnect out"=w591:T1)  [unwired: 5 in]
                      }
                      n148 = call "Out_On_F5xxx.vi"("DriverConnect in"=w567, "Model"=w561, "Output Signal Auto ON"=w542, "error in"=w566, "Error Code"=w544, "Driver Name"=w543) -> ("error out"=w538:T13)  [unwired: 8 in, 1 out]
                    }
                  }
                }
                frame 0, 3 {
                  # "F"
                  # "U"
                  n149 = Equal?(x=w628, y="AUX") -> (x = y?=w607:bool)
                  n150 = call "Out_Off_F5xxx.vi"("Driver Name"=w626, "SwitchOFF"=w629, "Error Code"=w627, "Model"=w631, "DriverConnect in"=w624) -> ("error out"=w605:T13, "DriverConnect out"=w608:T1)  [unwired: 5 in]
                  n151 = case shown="False" w607 {
                    tunnel: [w634 w639] -> w609
                    tunnel: w608 -> [w634 w640]
                    tunnel: ["%.;OUT %#e V," ("format string") w636] -> w606
                    tunnel: w605 -> [w632 w641]
                    tunnel: [w632 w638] -> w604
                    frame False {
                    }
                    frame True {
                      n152 = call "MLLF_WriteToBuffer.vi"("String"="OUT?" ("y"), "error in"=w641, "DriverConnect in"=w640) -> ("error out"=w642:T13, "DriverConnect out"=w643:T1)  [unwired: 5 in]
                      n153 = call "MLLF_ReadBuffer.vi"("Error In"=w642, "DriverConnect in"=w643) -> ("Error Out"=w646:errorcluster, "DriverConnect out"=w639:T1, "String"=w645:string)  [unwired: 6 in]
                      n154 = call "F5000_Find_V.vi"("Error In"=w646, "String in"=w645) -> ("Error Out"=w638:errorcluster, "String out"=w635:string)  [unwired: 8 in]
                      n155 = Concatenate Strings(w635, ", %.;%#e V," ("format string")) -> (w636:string)
                    }
                  }
                  n156 = call "MLLF_FormatStringValue.vi"("error in"=w604, "String Value"=w603, "Format"=w606) -> ("error out"=w613:T13, "String Value Formated"=w618:T14)  [unwired: 6 in, 1 out]
                  n157 = call "MLLF_ParameterSelect.vi"("Command to equipment"=string[] ["SINE", "SQUARE", "TRI", "TRUNCS", "NONE", "SINE"] ("Parameters"), "Names"=string[][] [["SIN", "SINE"], ["SQU", "SQUARE"], ["TRI", "TRIANGLE"], ["TRUNCS", "TRUNCSIN"], ["NONE", "NO"], ["", ""]], "Input"=w601, "Error In"=w613, "Command"=w630, "Driver Name"=w626, "Error Code"=w627) -> ("Choice"=w611:string, "Error Out"=w612:errorcluster)  [unwired: 7 in]
                  n158 = case shown="0, Default" w631 {
                    tunnel: [w647 "%.;%#e HZ;" ("format string")] -> w617
                    tunnel: w611 -> [w648 _]
                    frame 0, Default {
                      n159 = Concatenate Strings("%.;%#e HZ; WAVE " ("format string"), w648, ";" ("format string")) -> (w647:string)
                    }
                    frame 2, 3 {
                    }
                  }
                  n160 = Concatenate Strings(w618, w617) -> (w614:string)
                  n161 = call "MLLF_FormatStringValue.vi"("error in"=w612, "String Value"=w602, "Format"=w614) -> ("error out"=w620:T13, "String Value Formated"=w619:T14)  [unwired: 6 in, 1 out]
                  n162 = for {
                    N: 3 -> [_]
                    tunnel: w609 -> [w661]
                    tunnel: w620 -> [w660]
                    tunnel: w619 -> [w659]
                    tunnel: [w653] -> w622
                    tunnel: [w654] -> w621
                    tunnel: w627 -> [w656]
                    tunnel: w626 -> [w655]
                    tunnel: w631 -> [w652]
                    stop <- w654 continue-if-true
                    n163 = call "MLLF_WriteToBuffer.vi"("String"=w659, "error in"=w660, "DriverConnect in"=w661) -> ("error out"=w658:T13, "DriverConnect out"=w657:T1)  [unwired: 5 in]
                    n164 = call "F5xxx_ESR_check.vi"("Driver Name"=w655, "Error Code"=w656, "Model"=w652, "error in"=w658, "DriverConnect in"=w657) -> ("error out"=w654:T13, "DriverConnect out"=w653:T1)  [unwired: 5 in]
                  }
                  n165 = call "Out_On_F5xxx.vi"("DriverConnect in"=w622, "Model"=w631, "Output Signal Auto ON"=w625, "error in"=w621, "Error Code"=w627, "Driver Name"=w626) -> ("error out"=w600:T13)  [unwired: 8 in, 1 out]
                }
                frame 6 {
                  # "F"
                  # "U"
                  n166 = Equal?(x=w685, y="AUX") -> (x = y?=w669:bool)
                  n167 = call "Out_Off_F5xxx.vi"("Driver Name"=w683, "SwitchOFF"=w686, "Error Code"=w684, "Model"=w687, "DriverConnect in"=w681) -> ("error out"=w667:T13, "DriverConnect out"=w670:T1)  [unwired: 5 in]
                  n168 = case shown="False" w669 {
                    tunnel: [w690 w695] -> w671
                    tunnel: w670 -> [w690 w696]
                    tunnel: ["%.;OUT %#e V," ("format string") w692] -> w668
                    tunnel: w667 -> [w688 w697]
                    tunnel: [w688 w694] -> w666
                    frame False {
                    }
                    frame True {
                      n169 = call "MLLF_WriteToBuffer.vi"("String"="OUT?" ("y"), "error in"=w697, "DriverConnect in"=w696) -> ("error out"=w698:T13, "DriverConnect out"=w699:T1)  [unwired: 5 in]
                      n170 = call "MLLF_ReadBuffer.vi"("Error In"=w698, "DriverConnect in"=w699) -> ("Error Out"=w702:errorcluster, "DriverConnect out"=w695:T1, "String"=w701:string)  [unwired: 6 in]
                      n171 = call "F5000_Find_V.vi"("Error In"=w702, "String in"=w701) -> ("Error Out"=w694:errorcluster, "String out"=w691:string)  [unwired: 8 in]
                      n172 = Concatenate Strings(w691, ", %.;%#e V," ("format string")) -> (w692:string)
                    }
                  }
                  n173 = call "MLLF_FormatStringValue.vi"("error in"=w666, "String Value"=w664, "Format"=w668) -> ("error out"=w665:T13, "String Value Formated"=w675:T14)  [unwired: 6 in, 1 out]
                  n174 = case shown="0, Default" w687 {
                    tunnel: [w703 "%.;%#e HZ;" ("format string")] -> w674
                    frame 0, Default {
                      n175 = Concatenate Strings("%.;%#e HZ;" ("format string"), ";" ("format string")) -> (w703:string)
                    }
                    frame 2, 3 {
                    }
                  }
                  n176 = Concatenate Strings(w675, w674) -> (w673:string)
                  n177 = call "MLLF_FormatStringValue.vi"("error in"=w665, "String Value"=w663, "Format"=w673) -> ("error out"=w677:T13, "String Value Formated"=w676:T14)  [unwired: 6 in, 1 out]
                  n178 = for {
                    N: 3 -> [_]
                    tunnel: w671 -> [w716]
                    tunnel: w677 -> [w715]
                    tunnel: w676 -> [w714]
                    tunnel: [w708] -> w679
                    tunnel: [w709] -> w678
                    tunnel: w684 -> [w711]
                    tunnel: w683 -> [w710]
                    tunnel: w687 -> [w707]
                    stop <- w709 continue-if-true
                    n179 = call "MLLF_WriteToBuffer.vi"("String"=w714, "error in"=w715, "DriverConnect in"=w716) -> ("error out"=w713:T13, "DriverConnect out"=w712:T1)  [unwired: 5 in]
                    n180 = call "F5xxx_ESR_check.vi"("Driver Name"=w710, "Error Code"=w711, "Model"=w707, "error in"=w713, "DriverConnect in"=w712) -> ("error out"=w709:T13, "DriverConnect out"=w708:T1)  [unwired: 5 in]
                  }
                  n181 = call "Out_On_F5xxx.vi"("DriverConnect in"=w679, "Model"=w687, "Output Signal Auto ON"=w682, "error in"=w678, "Error Code"=w684, "Driver Name"=w683) -> ("error out"=w662:T13)  [unwired: 8 in, 1 out]
                }
              }
            }
            frame "PowerDC" {
              # "PowerDC=10 0,5"
              n182 = call "Out_Off_F5xxx.vi"("Driver Name"=w732, "SwitchOFF"=w730, "Error Code"=w731, "Model"=w720, "DriverConnect in"=w739) -> ("error out"=w721:T13, "DriverConnect out"=w729:T1)  [unwired: 5 in]
              n183 = call "MLLF_FormatStringValue.vi"("error in"=w721, "String Value"=w718, "Format"="OUT %.;%#e V" ("format string")) -> ("error out"=w727:T13, "String Value Formated"=w733:T14)  [unwired: 6 in, 1 out]
              n184 = case shown="0, Default" w720 {
                tunnel: [", 0 HZ; WAVE NONE;" ("format string") ", 0 HZ;" ("format string")] -> w724
                frame 0, Default {
                }
                frame 2, 3 {
                }
              }
              n185 = call "MLLF_FormatStringValue.vi"("error in"=w727, "String Value"=w717, "Format"=",  %.;%#e A" ("format")) -> ("error out"=w725:T13, "String Value Formated"=w723:T14)  [unwired: 6 in, 1 out]
              n186 = Concatenate Strings(w733, w723, w724) -> (w726:string)
              n187 = for {
                N: 2 -> [_]
                tunnel: w729 -> [w751]
                tunnel: w725 -> [w750]
                tunnel: w726 -> [w749]
                tunnel: [w743] -> w736
                tunnel: [w744] -> w735
                tunnel: w731 -> [w746]
                tunnel: w732 -> [w745]
                tunnel: w720 -> [w742]
                stop <- w744 continue-if-true
                n188 = call "MLLF_WriteToBuffer.vi"("String"=w749, "error in"=w750, "DriverConnect in"=w751) -> ("error out"=w748:T13, "DriverConnect out"=w747:T1)  [unwired: 5 in]
                n189 = call "F5xxx_ESR_check.vi"("Driver Name"=w745, "Error Code"=w746, "Model"=w742, "error in"=w748, "DriverConnect in"=w747) -> ("error out"=w744:T13, "DriverConnect out"=w743:T1)  [unwired: 5 in]
              }
              n190 = call "Out_On_F5xxx.vi"("DriverConnect in"=w736, "Model"=w720, "Output Signal Auto ON"=w719, "error in"=w735, "Error Code"=w731, "Driver Name"=w732) -> ("error out"=w734:T13)  [unwired: 8 in, 1 out]
            }
            frame "PHASE" {
              # "PHASE=90"
              n191 = call "MLLF_FormatStringValue.vi"("String Value"=w752, "Format"="PHASE %.;%#e DEG" ("format string")) -> ("error out"=w754:T13, "String Value Formated"=w756:T14)  [unwired: 7 in, 1 out]
              n192 = for {
                N: 2 -> [_]
                tunnel: w755 -> [w772]
                tunnel: w756 -> [w771]
                tunnel: [w765] -> _
                tunnel: [w766] -> w753
                tunnel: w759 -> [w768]
                tunnel: w760 -> [w767]
                tunnel: w757 -> [w764]
                tunnel: w754 -> [w763]
                stop <- w766 continue-if-true
                n193 = call "MLLF_WriteToBuffer.vi"("String"=w771, "error in"=w763, "DriverConnect in"=w772) -> ("error out"=w770:T13, "DriverConnect out"=w769:T1)  [unwired: 5 in]
                n194 = call "F5xxx_ESR_check.vi"("Driver Name"=w767, "Error Code"=w768, "Model"=w764, "error in"=w770, "DriverConnect in"=w769) -> ("error out"=w766:T13, "DriverConnect out"=w765:T1)  [unwired: 5 in]
              }
            }
            frame "PowerAC" {
              # "PowerAC=10 0,5 50"
              n195 = call "Out_Off_F5xxx.vi"("Driver Name"=w791, "SwitchOFF"=w789, "Error Code"=w790, "Model"=w781, "DriverConnect in"=w798) -> ("error out"=w782:T13, "DriverConnect out"=w788:T1)  [unwired: 5 in]
              n196 = call "MLLF_FormatStringValue.vi"("error in"=w782, "String Value"=w775, "Format"="OUT %.;%#e V" ("format string")) -> ("error out"=w786:T13, "String Value Formated"=w792:T14)  [unwired: 6 in, 1 out]
              n197 = case shown="0, Default" w781 {
                tunnel: [", %.;%#e HZ; WAVE SINE;" ("format string") ", %.;%#e HZ;" ("format string")] -> w778
                frame 0, Default {
                }
                frame 2, 3 {
                }
              }
              n198 = call "MLLF_FormatStringValue.vi"("error in"=w786, "String Value"=w774, "Format"=", %.;%#e A" ("format")) -> ("error out"=w780:T13, "String Value Formated"=w784:T14)  [unwired: 6 in, 1 out]
              n199 = call "MLLF_FormatStringValue.vi"("error in"=w780, "String Value"=w773, "Format"=w778) -> ("error out"=w779:T13, "String Value Formated"=w777:T14)  [unwired: 6 in, 1 out]
              n200 = Concatenate Strings(w792, w784, w777) -> (w785:string)
              n201 = for {
                N: 2 -> [_]
                tunnel: w788 -> [w810]
                tunnel: w779 -> [w809]
                tunnel: w785 -> [w808]
                tunnel: [w802] -> w795
                tunnel: [w803] -> w794
                tunnel: w790 -> [w805]
                tunnel: w791 -> [w804]
                tunnel: w781 -> [w801]
                stop <- w803 continue-if-true
                n202 = call "MLLF_WriteToBuffer.vi"("String"=w808, "error in"=w809, "DriverConnect in"=w810) -> ("error out"=w807:T13, "DriverConnect out"=w806:T1)  [unwired: 5 in]
                n203 = call "F5xxx_ESR_check.vi"("Driver Name"=w804, "Error Code"=w805, "Model"=w801, "error in"=w807, "DriverConnect in"=w806) -> ("error out"=w803:T13, "DriverConnect out"=w802:T1)  [unwired: 5 in]
              }
              n204 = call "Out_On_F5xxx.vi"("DriverConnect in"=w795, "Model"=w781, "Output Signal Auto ON"=w776, "error in"=w794, "Error Code"=w790, "Driver Name"=w791) -> ("error out"=w793:T13)  [unwired: 8 in, 1 out]
            }
            frame "IDC" {
              # "IDC= 250m"
              # "CUR_POST AUX; OUT 0.15A, 0 HZ; WAVE NONE;"
              # "I"
              n205 = call "Out_Off_F5xxx.vi"("Driver Name"=w814, "SwitchOFF"=w818, "Error Code"=w815, "Model"=w820, "DriverConnect in"=w831) -> ("error out"=w819:T13, "DriverConnect out"=w830:T1)  [unwired: 5 in]
              n206 = case shown="3, 6" w820 {
                tunnel: ["%.;OUT %#e A, 0 HZ; WAVE NONE;" ("format string") "%.;OUT %#e A, 0 HZ;" ("format string")] -> w821
                frame 0, Default {
                }
                frame 3, 6 {
                }
              }
              n207 = call "MLLF_FormatStringValue.vi"("error in"=w819, "String Value"=w813, "Format"=w821) -> ("error out"=w817:T13, "String Value Formated"=w824:T14)  [unwired: 6 in, 1 out]
              n208 = Format Into String(format string="CUR_POST %s; %s", error in=w817, w816, w824) -> (resulting string=w825:string, error out=w823:errorcluster)  [unwired: 1 in]
              n209 = for {
                N: 2 -> [_]
                tunnel: w830 -> [w843]
                tunnel: w823 -> [w842]
                tunnel: w825 -> [w841]
                tunnel: [w836] -> w827
                tunnel: [w835] -> w822
                tunnel: w815 -> [w838]
                tunnel: w814 -> [w837]
                tunnel: w820 -> [w834]
                stop <- w835 continue-if-true
                n210 = call "MLLF_WriteToBuffer.vi"("String"=w841, "error in"=w842, "DriverConnect in"=w843) -> ("error out"=w840:T13, "DriverConnect out"=w839:T1)  [unwired: 5 in]
                n211 = call "F5xxx_ESR_check.vi"("Driver Name"=w837, "Error Code"=w838, "Model"=w834, "error in"=w840, "DriverConnect in"=w839) -> ("error out"=w835:T13, "DriverConnect out"=w836:T1)  [unwired: 5 in]
              }
              n212 = call "Out_On_F5xxx.vi"("DriverConnect in"=w827, "Model"=w820, "Output Signal Auto ON"=w812, "error in"=w822, "Error Code"=w815, "Driver Name"=w814) -> ("error out"=w811:T13)  [unwired: 8 in, 1 out]
            }
            frame "IAC" {
              # "IAC=200m 100"
              # "CUR_POST AUX; OUT 0.001A, 50HZ; WAVE SINE;"
              n213 = case shown="Default" w847 {
                tunnel: w855 -> [w870 w970]
                tunnel: w854 -> [w869 w953]
                tunnel: w853 -> [w868 w969]
                tunnel: w852 -> [w867 w968]
                tunnel: [w866 w957] -> w844
                tunnel: w851 -> [w865 _]
                tunnel: w850 -> [w864 w960]
                tunnel: w849 -> [w863 w952]
                tunnel: w848 -> [w861 w966]
                tunnel: w847 -> [w860 w967]
                tunnel: w846 -> [w858 _]
                tunnel: w845 -> [w857 w959]
                frame Default {
                  n214 = case shown="True" w858 {
                    tunnel: [w872 w875] -> w862
                    tunnel: w861 -> [w872 w874]
                    tunnel: ["OFF" ("String") w873] -> w859
                    frame False {
                    }
                    frame True {
                      n215 = call "MLLF_WriteToBuffer.vi"("String"="PQ?", "DriverConnect in"=w874) -> ("error out"=w878:T13, "DriverConnect out"=w877:T1)  [unwired: 6 in]
                      n216 = call "MLLF_ReadBuffer.vi"("Error In"=w878, "DriverConnect in"=w877) -> ("DriverConnect out"=w875:T1, "String"=w873:string)  [unwired: 6 in, 1 out]
                    }
                  }
                  n217 = case shown="\"CH\"" w859 {
                    tunnel: w862 -> [w902 w938]
                    tunnel: w860 -> [w890 w926]
                    tunnel: w870 -> [w888 w924]
                    tunnel: w869 -> [w886 w922]
                    tunnel: w868 -> [w885 w921]
                    tunnel: w867 -> [w884 w920]
                    tunnel: [w879 w915] -> w866
                    tunnel: w865 -> [_ _]
                    tunnel: w864 -> [w882 w918]
                    tunnel: w863 -> [w883 w919]
                    tunnel: w857 -> [w881 w917]
                    frame "OFF", Default {
                      # "I"
                      n218 = call "Out_Off_F5xxx.vi"("Driver Name"=w884, "SwitchOFF"=w888, "Error Code"=w885, "Model"=w890, "DriverConnect in"=w902) -> ("error out"=w897:T13, "DriverConnect out"=w901:T1)  [unwired: 5 in]
                      n219 = call "MLLF_FormatStringValue.vi"("error in"=w897, "String Value"=w882, "Format"="%.;OUT %#e A" ("format string")) -> ("error out"=w896:T13, "String Value Formated"=w893:T14)  [unwired: 6 in, 1 out]
                      n220 = case shown="3, 6" w890 {
                        tunnel: ["%.;%#e HZ; WAVE SINE;" ("format string") "%.;%#e HZ;" ("format string")] -> w891
                        frame 0, Default {
                        }
                        frame 3, 6 {
                        }
                      }
                      n221 = call "MLLF_FormatStringValue.vi"("error in"=w896, "String Value"=w881, "Format"=w891) -> ("error out"=w887:T13, "String Value Formated"=w892:T14)  [unwired: 6 in, 1 out]
                      n222 = Format Into String(format string="CUR_POST %s; %s, %s", error in=w887, w886, w893, w892) -> (resulting string=w880:string, error out=w894:errorcluster)  [unwired: 1 in]
                      n223 = for {
                        N: 2 -> [_]
                        tunnel: w901 -> [w914]
                        tunnel: w894 -> [w913]
                        tunnel: w880 -> [w912]
                        tunnel: [w909] -> w899
                        tunnel: [w908] -> w889
                        tunnel: w885 -> [w907]
                        tunnel: w884 -> [w906]
                        tunnel: w890 -> [w905]
                        stop <- w908 continue-if-true
                        n224 = call "MLLF_WriteToBuffer.vi"("String"=w912, "error in"=w913, "DriverConnect in"=w914) -> ("error out"=w911:T13, "DriverConnect out"=w910:T1)  [unwired: 5 in]
                        n225 = call "F5xxx_ESR_check.vi"("Driver Name"=w906, "Error Code"=w907, "Model"=w905, "error in"=w911, "DriverConnect in"=w910) -> ("error out"=w908:T13, "DriverConnect out"=w909:T1)  [unwired: 5 in]
                      }
                      n226 = call "Out_On_F5xxx.vi"("DriverConnect in"=w899, "Model"=w890, "Output Signal Auto ON"=w883, "error in"=w889, "Error Code"=w885, "Driver Name"=w884) -> ("error out"=w879:T13)  [unwired: 8 in, 1 out]
                    }
                    frame "CH" {
                      # "I"
                      n227 = call "Out_Off_F5xxx.vi"("Driver Name"=w920, "SwitchOFF"=w924, "Error Code"=w921, "Model"=w926, "DriverConnect in"=w938) -> ("error out"=w933:T13, "DriverConnect out"=w937:T1)  [unwired: 5 in]
                      n228 = call "MLLF_FormatStringValue.vi"("error in"=w933, "String Value"=w918, "Format"="%.;OUT %#e A" ("format string")) -> ("error out"=w932:T13, "String Value Formated"=w929:T14)  [unwired: 6 in, 1 out]
                      n229 = case shown="0, Default" w926 {
                        tunnel: ["%.;%#e HZ;" ("format string") "%.;%#e HZ;" ("format string")] -> w927
                        frame 0, Default {
                        }
                        frame 2, 3 {
                        }
                      }
                      n230 = call "MLLF_FormatStringValue.vi"("error in"=w932, "String Value"=w917, "Format"=w927) -> ("error out"=w923:T13, "String Value Formated"=w928:T14)  [unwired: 6 in, 1 out]
                      n231 = Format Into String(format string="CUR_POST %s; %s, %s", error in=w923, w922, w929, w928) -> (resulting string=w916:string, error out=w930:errorcluster)  [unwired: 1 in]
                      n232 = for {
                        N: 2 -> [_]
                        tunnel: w937 -> [w950]
                        tunnel: w930 -> [w949]
                        tunnel: w916 -> [w948]
                        tunnel: [w945] -> w935
                        tunnel: [w944] -> w925
                        tunnel: w921 -> [w943]
                        tunnel: w920 -> [w942]
                        tunnel: w926 -> [w941]
                        stop <- w944 continue-if-true
                        n233 = call "MLLF_WriteToBuffer.vi"("String"=w948, "error in"=w949, "DriverConnect in"=w950) -> ("error out"=w947:T13, "DriverConnect out"=w946:T1)  [unwired: 5 in]
                        n234 = call "F5xxx_ESR_check.vi"("Driver Name"=w942, "Error Code"=w943, "Model"=w941, "error in"=w947, "DriverConnect in"=w946) -> ("error out"=w944:T13, "DriverConnect out"=w945:T1)  [unwired: 5 in]
                      }
                      n235 = call "Out_On_F5xxx.vi"("DriverConnect in"=w935, "Model"=w926, "Output Signal Auto ON"=w919, "error in"=w925, "Error Code"=w921, "Driver Name"=w920) -> ("error out"=w915:T13)  [unwired: 8 in, 1 out]
                    }
                  }
                }
                frame 0, 3, 6 {
                  n236 = call "Out_Off_F5xxx.vi"("Driver Name"=w968, "SwitchOFF"=w970, "Error Code"=w969, "Model"=w967, "DriverConnect in"=w966) -> ("error out"=w963:T13, "DriverConnect out"=w956:T1)  [unwired: 5 in]
                  n237 = stacked-sequence {
                    tunnel: w953 -> [w984 _]
                    tunnel: w967 -> [w971 _]
                    tunnel: w963 -> [w982 _]
                    tunnel: [w979 _] -> w962
                    tunnel: w960 -> [w974 _]
                    tunnel: w959 -> [w973 _]
                    tunnel: [w972 _] -> w958
                    tunnel: w956 -> [_ w988]
                    tunnel: [_ w988] -> w955
                    tunnel: [w971 _] -> w954
                    tunnel: w952 -> [_ w987]
                    tunnel: [_ w987] -> w951
                    frame #0 {
                      # "I"
                      n238 = call "MLLF_FormatStringValue.vi"("error in"=w982, "String Value"=w974, "Format"="%.;OUT %#e A" ("format string")) -> ("error out"=w981:T13, "String Value Formated"=w978:T14)  [unwired: 6 in, 1 out]
                      n239 = case shown="0, Default" w971 {
                        tunnel: ["%.;%#e HZ; WAVE SINE;" ("format string") "%.;%#e HZ;" ("format string")] -> w976
                        frame 0, Default {
                        }
                        frame 3, 6 {
                        }
                      }
                      n240 = call "MLLF_FormatStringValue.vi"("error in"=w981, "String Value"=w973, "Format"=w976) -> ("error out"=w975:T13, "String Value Formated"=w977:T14)  [unwired: 6 in, 1 out]
                      n241 = Format Into String(format string="CUR_POST %s; %s, %s", error in=w975, w984, w978, w977) -> (resulting string=w972:string, error out=w979:errorcluster)  [unwired: 1 in]
                    }
                    frame #1 {
                    }
                  }
                  n242 = for {
                    N: 2 -> [_]
                    tunnel: w955 -> [w998]
                    tunnel: w962 -> [w997]
                    tunnel: w958 -> [w996]
                    tunnel: [w993] -> w964
                    tunnel: [w992] -> w961
                    tunnel: w969 -> [w991]
                    tunnel: w968 -> [w990]
                    tunnel: w954 -> [w989]
                    stop <- w992 continue-if-true
                    n243 = call "MLLF_WriteToBuffer.vi"("String"=w996, "error in"=w997, "DriverConnect in"=w998) -> ("error out"=w995:T13, "DriverConnect out"=w994:T1)  [unwired: 5 in]
                    n244 = call "F5xxx_ESR_check.vi"("Driver Name"=w990, "Error Code"=w991, "Model"=w989, "error in"=w995, "DriverConnect in"=w994) -> ("error out"=w992:T13, "DriverConnect out"=w993:T1)  [unwired: 5 in]
                  }
                  n245 = call "Out_On_F5xxx.vi"("DriverConnect in"=w964, "Model"=w954, "Output Signal Auto ON"=w951, "error in"=w961, "Error Code"=w969, "Driver Name"=w968) -> ("error out"=w957:T13)  [unwired: 8 in, 1 out]
                }
              }
            }
            frame "R", "RES" {
              # "OUT 100kOHM; ZCOMP NONE;"
              # "R=100k"
              n246 = call "Out_Off_F5xxx.vi"("Driver Name"=w1016, "SwitchOFF"=w1018, "Error Code"=w1017, "Model"=w1012, "DriverConnect in"=w1021) -> ("error out"=w1004:T13, "DriverConnect out"=w1010:T1)  [unwired: 5 in]
              n247 = call "MLLF_FormatStringValue.vi"("error in"=w1004, "String Value"=w1014, "Format"="%.;OUT %#e OHM; " ("format string")) -> ("error out"=w1002:T13, "String Value Formated"=w1000:T14)  [unwired: 6 in, 1 out]
              n248 = call "F5xxx_ZCOMP.vi"("Parameter"=w1015, "Conn"=w1019, "Model"=w1012) -> ("Error Query"=w1005:string)  [unwired: 8 in]
              n249 = Format Into String(format string="%s  %s;", error in=w1002, w1000, w1005) -> (resulting string=w1009:string, error out=w1001:errorcluster)  [unwired: 1 in]
              n250 = for {
                N: 2 -> [_]
                tunnel: w1010 -> [w1031]
                tunnel: w1001 -> [w1030]
                tunnel: w1009 -> [w1029]
                tunnel: [w1024] -> w1007
                tunnel: [w1023] -> w1006
                tunnel: w1017 -> [w1026]
                tunnel: w1016 -> [w1025]
                tunnel: w1012 -> [w1022]
                stop <- w1023 continue-if-true
                n251 = call "MLLF_WriteToBuffer.vi"("String"=w1029, "error in"=w1030, "DriverConnect in"=w1031) -> ("error out"=w1028:T13, "DriverConnect out"=w1027:T1)  [unwired: 5 in]
                n252 = call "F5xxx_ESR_check.vi"("Driver Name"=w1025, "Error Code"=w1026, "Model"=w1022, "error in"=w1028, "DriverConnect in"=w1027) -> ("error out"=w1023:T13, "DriverConnect out"=w1024:T1)  [unwired: 5 in]
              }
              n253 = call "Out_On_F5xxx.vi"("DriverConnect in"=w1007, "Model"=w1012, "Output Signal Auto ON"=w1013, "error in"=w1006, "Error Code"=w1017, "Driver Name"=w1016) -> ("error out"=w999:T13)  [unwired: 8 in, 1 out]
            }
            frame "C" {
              # "C=10n"
              # "OUT 10UF; ZCOMP NONE;"
              n254 = call "Out_Off_F5xxx.vi"("Driver Name"=w1043, "SwitchOFF"=w1033, "Error Code"=w1044, "Model"=w1036, "DriverConnect in"=w1053) -> ("error out"=w1041:T13, "DriverConnect out"=w1051:T1)  [unwired: 5 in]
              n255 = call "MLLF_FormatStringValue.vi"("error in"=w1041, "String Value"=w1042, "Format"="%.;OUT %#e F;" ("format string")) -> ("error out"=w1039:T13, "String Value Formated"=w1038:T14)  [unwired: 6 in, 1 out]
              n256 = call "F5xxx_ZCOMP.vi"("Parameter"=w1034, "Conn"=w1037, "Model"=w1036) -> ("Error Query"=w1035:string)  [unwired: 8 in]
              n257 = Format Into String(format string="%s  %s;", error in=w1039, w1038, w1035) -> (resulting string=w1050:string)  [unwired: 1 in, 1 out]
              n258 = for {
                N: 2 -> [_]
                tunnel: w1051 -> [w1062]
                tunnel: w1050 -> [w1061]
                tunnel: [w1056] -> w1048
                tunnel: [w1055] -> w1047
                tunnel: w1044 -> [w1058]
                tunnel: w1043 -> [w1057]
                tunnel: w1036 -> [w1054]
                stop <- w1055 continue-if-true
                n259 = call "MLLF_WriteToBuffer.vi"("String"=w1061, "DriverConnect in"=w1062) -> ("error out"=w1060:T13, "DriverConnect out"=w1059:T1)  [unwired: 6 in]
                n260 = call "F5xxx_ESR_check.vi"("Driver Name"=w1057, "Error Code"=w1058, "Model"=w1054, "error in"=w1060, "DriverConnect in"=w1059) -> ("error out"=w1055:T13, "DriverConnect out"=w1056:T1)  [unwired: 5 in]
              }
              n261 = call "Out_On_F5xxx.vi"("DriverConnect in"=w1048, "Model"=w1036, "Output Signal Auto ON"=w1032, "error in"=w1047, "Error Code"=w1044, "Driver Name"=w1043) -> ("error out"=w1046:T13)  [unwired: 8 in, 1 out]
            }
            frame "TC" {
              # "type"
              # "TC=30 \tJ"
              # "TSENS_TYPE TC; TC_TYPE K; OUT 1CEL;"
              n262 = call "Out_Off_F5xxx.vi"("Driver Name"=w1075, "SwitchOFF"=w1068, "Error Code"=w1074, "Model"=w1070, "DriverConnect in"=w1087) -> ("error out"=w1073:T13, "DriverConnect out"=w1085:T1)  [unwired: 5 in]
              n263 = call "F5xxx_ZCOMP.vi"("Parameter"=w1071, "Conn"=w1072, "Model"=w1070) -> ("Error Query"=w1069:string)  [unwired: 8 in]
              n264 = call "MLLF_FormatStringValue.vi"("error in"=w1073, "String Value"=w1064, "Format"="%.;OUT %#e CEL" ("format string")) -> ("error out"=w1067:T13, "String Value Formated"=w1078:T14)  [unwired: 6 in, 1 out]
              n265 = To Upper Case(1:w1063) -> (0:w1066:string)
              n266 = Format Into String(format string="%.;TSENS_TYPE TC; TC_TYPE %s;  %s; %s", error in=w1067, w1066, w1078, w1069) -> (resulting string=w1084:string, error out=w1076:errorcluster)  [unwired: 1 in]
              n267 = for {
                N: 2 -> [_]
                tunnel: w1085 -> [w1097]
                tunnel: w1084 -> [w1096]
                tunnel: [w1091] -> w1082
                tunnel: [w1090] -> w1077
                tunnel: w1074 -> [w1093]
                tunnel: w1075 -> [w1092]
                tunnel: w1070 -> [w1089]
                tunnel: w1076 -> [w1088]
                stop <- w1090 continue-if-true
                n268 = call "MLLF_WriteToBuffer.vi"("String"=w1096, "error in"=w1088, "DriverConnect in"=w1097) -> ("error out"=w1095:T13, "DriverConnect out"=w1094:T1)  [unwired: 5 in]
                n269 = call "F5xxx_ESR_check.vi"("Driver Name"=w1092, "Error Code"=w1093, "Model"=w1089, "error in"=w1095, "DriverConnect in"=w1094) -> ("error out"=w1090:T13, "DriverConnect out"=w1091:T1)  [unwired: 5 in]
              }
              n270 = call "Out_On_F5xxx.vi"("DriverConnect in"=w1082, "Model"=w1070, "Output Signal Auto ON"=w1065, "error in"=w1077, "Error Code"=w1074, "Driver Name"=w1075) -> ("error out"=w1081:T13)  [unwired: 8 in, 1 out]
            }
            frame "TF" {
              # "type"
              # "TF=-58 \tJ"
              # "TSENS_TYPE TC; TC_TYPE K; OUT 1CEL;"
              n271 = call "Out_Off_F5xxx.vi"("Driver Name"=w1110, "SwitchOFF"=w1103, "Error Code"=w1109, "Model"=w1105, "DriverConnect in"=w1122) -> ("error out"=w1108:T13, "DriverConnect out"=w1120:T1)  [unwired: 5 in]
              n272 = call "F5xxx_ZCOMP.vi"("Parameter"=w1106, "Conn"=w1107, "Model"=w1105) -> ("Error Query"=w1104:string)  [unwired: 8 in]
              n273 = call "MLLF_FormatStringValue.vi"("error in"=w1108, "String Value"=w1099, "Format"="%.;OUT %#e FAR" ("format string")) -> ("error out"=w1102:T13, "String Value Formated"=w1113:T14)  [unwired: 6 in, 1 out]
              n274 = To Upper Case(1:w1098) -> (0:w1101:string)
              n275 = Format Into String(format string="%.;TSENS_TYPE TC; TC_TYPE %s;  %s; %s", error in=w1102, w1101, w1113, w1104) -> (resulting string=w1119:string, error out=w1111:errorcluster)  [unwired: 1 in]
              n276 = for {
                N: 2 -> [_]
                tunnel: w1120 -> [w1132]
                tunnel: w1119 -> [w1131]
                tunnel: [w1126] -> w1117
                tunnel: [w1125] -> w1112
                tunnel: w1109 -> [w1128]
                tunnel: w1110 -> [w1127]
                tunnel: w1105 -> [w1124]
                tunnel: w1111 -> [w1123]
                stop <- w1125 continue-if-true
                n277 = call "MLLF_WriteToBuffer.vi"("String"=w1131, "error in"=w1123, "DriverConnect in"=w1132) -> ("error out"=w1130:T13, "DriverConnect out"=w1129:T1)  [unwired: 5 in]
                n278 = call "F5xxx_ESR_check.vi"("Driver Name"=w1127, "Error Code"=w1128, "Model"=w1124, "error in"=w1130, "DriverConnect in"=w1129) -> ("error out"=w1125:T13, "DriverConnect out"=w1126:T1)  [unwired: 5 in]
              }
              n279 = call "Out_On_F5xxx.vi"("DriverConnect in"=w1117, "Model"=w1105, "Output Signal Auto ON"=w1100, "error in"=w1112, "Error Code"=w1109, "Driver Name"=w1110) -> ("error out"=w1116:T13)  [unwired: 8 in, 1 out]
            }
            frame "TC_Ref_Point" {
              # "TC_Ref_Point=20\nTC_Ref_Point=int"
              n280 = case shown="\"False\", Default" w1134 {
                selector: w1134 -> [w1144 _]
                tunnel: [w1145 _] -> w1136
                tunnel: [w1143 "TC_REF INT" ("format string")] -> w1133
                frame "False", Default {
                  n281 = call "MLLF_FormatStringValue.vi"("String Value"=w1144, "Format"="TC_REF EXT,  %#e CEL" ("format string")) -> ("error out"=w1145:T13, "String Value Formated"=w1143:T14)  [unwired: 7 in, 1 out]
                }
                frame "int", "internal" {
                }
              }
              n282 = for {
                N: 2 -> [_]
                tunnel: w1137 -> [w1157]
                tunnel: [w1152] -> _
                tunnel: [w1151] -> w1135
                tunnel: w1139 -> [w1154]
                tunnel: w1140 -> [w1153]
                tunnel: w1138 -> [w1150]
                tunnel: w1136 -> [w1149]
                tunnel: w1133 -> [w1148]
                stop <- w1151 continue-if-true
                n283 = call "MLLF_WriteToBuffer.vi"("String"=w1148, "error in"=w1149, "DriverConnect in"=w1157) -> ("error out"=w1156:T13, "DriverConnect out"=w1155:T1)  [unwired: 5 in]
                n284 = call "F5xxx_ESR_check.vi"("Driver Name"=w1153, "Error Code"=w1154, "Model"=w1150, "error in"=w1156, "DriverConnect in"=w1155) -> ("error out"=w1151:T13, "DriverConnect out"=w1152:T1)  [unwired: 5 in]
              }
            }
            frame "PRT", "RTD" {
              # "RTD=30\tPT385"
              # "type"
              # "TSENS_TYPE TC; TC_TYPE K; OUT 1CEL;"
              n285 = call "Out_Off_F5xxx.vi"("Driver Name"=w1170, "SwitchOFF"=w1163, "Error Code"=w1162, "Model"=w1165, "DriverConnect in"=w1181) -> ("error out"=w1168:T13, "DriverConnect out"=w1179:T1)  [unwired: 5 in]
              n286 = call "F5xxx_ZCOMP.vi"("Parameter"=w1166, "Conn"=w1167, "Model"=w1165) -> ("Error Query"=w1164:string)  [unwired: 8 in]
              n287 = call "MLLF_FormatStringValue.vi"("error in"=w1168, "Format"="%.;OUT %#e CEL" ("format string")) -> ("error out"=w1160:T13, "String Value Formated"=w1173:T14)  [unwired: 7 in, 1 out]
              n288 = To Upper Case(1:w1158) -> (0:w1169:string)
              n289 = Format Into String(format string="%.;TSENS_TYPE RTD; RTD_TYPE %s; %s; %s", error in=w1160, w1169, w1173, w1164) -> (resulting string=w1161:string, error out=w1171:errorcluster)  [unwired: 1 in]
              n290 = for {
                N: 2 -> [_]
                tunnel: w1179 -> [w1191]
                tunnel: w1161 -> [w1190]
                tunnel: [w1185] -> w1177
                tunnel: [w1184] -> w1172
                tunnel: w1162 -> [w1187]
                tunnel: w1170 -> [w1186]
                tunnel: w1165 -> [w1183]
                tunnel: w1171 -> [w1182]
                stop <- w1184 continue-if-true
                n291 = call "MLLF_WriteToBuffer.vi"("String"=w1190, "error in"=w1182, "DriverConnect in"=w1191) -> ("error out"=w1189:T13, "DriverConnect out"=w1188:T1)  [unwired: 5 in]
                n292 = call "F5xxx_ESR_check.vi"("Driver Name"=w1186, "Error Code"=w1187, "Model"=w1183, "error in"=w1189, "DriverConnect in"=w1188) -> ("error out"=w1184:T13, "DriverConnect out"=w1185:T1)  [unwired: 5 in]
              }
              n293 = call "Out_On_F5xxx.vi"("DriverConnect in"=w1177, "Model"=w1165, "Output Signal Auto ON"=w1159, "error in"=w1172, "Error Code"=w1162, "Driver Name"=w1170) -> ("error out"=w1176:T13)  [unwired: 8 in, 1 out]
            }
            frame "RTD_Standart" {
              # "RTD_Standart=TS90"
              # "scale"
              n294 = call "MLLF_ParameterSelect.vi"("Command to equipment"=string[] ["IPTS_68", "ITS_90"] ("Parameters"), "Names"=string[][] [["TS68", "TS68"], ["TS90", "TS90"]], "Input"=w1196, "Command"=w1192, "Driver Name"=w1199, "Error Code"=w1198) -> ("Choice"=w1194:string, "Error Out"=w1200:errorcluster)  [unwired: 8 in]
              n295 = Format Into String(format string="TEMP_STD %s", error in=w1200, w1194) -> (resulting string=w1206:string, error out=w1201:errorcluster)  [unwired: 1 in]
              n296 = for {
                N: 2 -> [_]
                tunnel: w1206 -> [w1217]
                tunnel: [w1212] -> _
                tunnel: [w1211] -> w1195
                tunnel: w1198 -> [w1214]
                tunnel: w1199 -> [w1213]
                tunnel: w1197 -> [w1210]
                tunnel: w1201 -> [w1209]
                tunnel: w1193 -> [w1208]
                stop <- w1211 continue-if-true
                n297 = call "MLLF_WriteToBuffer.vi"("String"=w1217, "error in"=w1209, "DriverConnect in"=w1208) -> ("error out"=w1216:T13, "DriverConnect out"=w1215:T1)  [unwired: 5 in]
                n298 = call "F5xxx_ESR_check.vi"("Driver Name"=w1213, "Error Code"=w1214, "Model"=w1210, "error in"=w1216, "DriverConnect in"=w1215) -> ("error out"=w1211:T13, "DriverConnect out"=w1212:T1)  [unwired: 5 in]
              }
            }
            frame "DPF" {
              # "DPF=1\nDPF=0,256"
              n299 = Concatenate Strings("DPF " ("string"), w1220) -> (w1219:string)
              n300 = for {
                N: 2 -> [_]
                tunnel: w1219 -> [w1236]
                tunnel: [w1231] -> _
                tunnel: [w1230] -> w1222
                tunnel: w1224 -> [w1233]
                tunnel: w1225 -> [w1232]
                tunnel: w1223 -> [w1229]
                tunnel: w1218 -> [w1228]
                stop <- w1230 continue-if-true
                n301 = call "MLLF_WriteToBuffer.vi"("String"=w1236, "DriverConnect in"=w1228) -> ("error out"=w1235:T13, "DriverConnect out"=w1234:T1)  [unwired: 6 in]
                n302 = call "F5xxx_ESR_check.vi"("Driver Name"=w1232, "Error Code"=w1233, "Model"=w1229, "error in"=w1235, "DriverConnect in"=w1234) -> ("error out"=w1230:T13, "DriverConnect out"=w1231:T1)  [unwired: 5 in]
              }
            }
            frame "<----SCOPE FUNCTIONS---->" {
            }
            frame "SCOPE_VDC", "SCOPEDC", "SCOPEVDC" {
              # "SCOPE VOLT; OUT -2V, 0 Hz"
              # "SCOPEDC=5"
              n303 = call "Out_Off_F5xxx.vi"("Driver Name"=w1251, "SwitchOFF"=w1239, "Error Code"=w1252, "Model"=w1240, "DriverConnect in"=w1259) -> ("error out"=w1248:T13, "DriverConnect out"=w1258:T1)  [unwired: 5 in]
              n304 = call "MLLF_FormatStringValue.vi"("error in"=w1248, "String Value"=w1249, "Format"="%.;OUT %#e V, 0 HZ;" ("format string")) -> ("error out"=w1247:T13, "String Value Formated"=w1245:T14)  [unwired: 6 in, 1 out]
              n305 = Format Into String(format string="%s; SCOPE VOLT; %s", initial string="OUT_IMP " ("format string"), error in=w1247, w1243, w1245) -> (resulting string=w1241:string, error out=w1242:errorcluster)
              n306 = for {
                N: 2 -> [_]
                tunnel: w1258 -> [w1269]
                tunnel: w1242 -> [w1268]
                tunnel: w1241 -> [w1267]
                tunnel: [w1262] -> w1255
                tunnel: [w1261] -> w1254
                tunnel: w1252 -> [w1266]
                tunnel: w1251 -> [w1265]
                tunnel: w1240 -> [w1260]
                stop <- w1261 continue-if-true
                n307 = call "MLLF_WriteToBuffer.vi"("String"=w1267, "error in"=w1268, "DriverConnect in"=w1269) -> ("error out"=w1264:T13, "DriverConnect out"=w1263:T1)  [unwired: 5 in]
                n308 = call "F5xxx_ESR_check.vi"("Driver Name"=w1265, "Error Code"=w1266, "Model"=w1260, "error in"=w1264, "DriverConnect in"=w1263) -> ("error out"=w1261:T13, "DriverConnect out"=w1262:T1)  [unwired: 5 in]
              }
              n309 = call "Out_On_F5xxx.vi"("DriverConnect in"=w1255, "Model"=w1240, "Output Signal Auto ON"=w1238, "error in"=w1254, "Error Code"=w1252, "Driver Name"=w1251) -> ("error out"=w1253:T13)  [unwired: 8 in, 1 out]
            }
            frame "SCOPE_SQU", "SCOPESQU" {
              # "ScopeSqu=20m"
              # "SCOPE VOLT; OUT -2V, 1 kHz"
              n310 = call "Out_Off_F5xxx.vi"("Driver Name"=w1283, "SwitchOFF"=w1271, "Error Code"=w1284, "Model"=w1272, "DriverConnect in"=w1291) -> ("error out"=w1280:T13, "DriverConnect out"=w1290:T1)  [unwired: 5 in]
              n311 = call "MLLF_FormatStringValue.vi"("error in"=w1280, "String Value"=w1281, "Format"="%.;OUT %#e V, 1 kHZ;" ("format string")) -> ("error out"=w1279:T13, "String Value Formated"=w1277:T14)  [unwired: 6 in, 1 out]
              n312 = Format Into String(format string="%s; SCOPE VOLT; %s", initial string="OUT_IMP " ("format string"), error in=w1279, w1275, w1277) -> (resulting string=w1273:string, error out=w1274:errorcluster)
              n313 = for {
                N: 2 -> [_]
                tunnel: w1290 -> [w1301]
                tunnel: w1274 -> [w1300]
                tunnel: w1273 -> [w1299]
                tunnel: [w1294] -> w1287
                tunnel: [w1293] -> w1286
                tunnel: w1284 -> [w1298]
                tunnel: w1283 -> [w1297]
                tunnel: w1272 -> [w1292]
                stop <- w1293 continue-if-true
                n314 = call "MLLF_WriteToBuffer.vi"("String"=w1299, "error in"=w1300, "DriverConnect in"=w1301) -> ("error out"=w1296:T13, "DriverConnect out"=w1295:T1)  [unwired: 5 in]
                n315 = call "F5xxx_ESR_check.vi"("Driver Name"=w1297, "Error Code"=w1298, "Model"=w1292, "error in"=w1296, "DriverConnect in"=w1295) -> ("error out"=w1293:T13, "DriverConnect out"=w1294:T1)  [unwired: 5 in]
              }
              n316 = call "Out_On_F5xxx.vi"("DriverConnect in"=w1287, "Model"=w1272, "Output Signal Auto ON"=w1270, "error in"=w1286, "Error Code"=w1284, "Driver Name"=w1283) -> ("error out"=w1285:T13)  [unwired: 8 in, 1 out]
            }
            frame "SCOPE_SIN", "SCOPESIN" {
              # "ScopeSIN=10M   30m"
              # "SCOPE LEVSINE; OUT 1V, 20 kHz"
              n317 = call "Out_Off_F5xxx.vi"("Driver Name"=w1319, "SwitchOFF"=w1305, "Error Code"=w1320, "Model"=w1307, "DriverConnect in"=w1327) -> ("error out"=w1317:T13, "DriverConnect out"=w1326:T1)  [unwired: 5 in]
              n318 = call "MLLF_FormatStringValue.vi"("error in"=w1317, "String Value"=w1302, "Format"="%.;OUT %#e V" ("format string")) -> ("error out"=w1309:T13, "String Value Formated"=w1315:T14)  [unwired: 6 in, 1 out]
              n319 = call "MLLF_FormatStringValue.vi"("error in"=w1309, "String Value"=w1303, "Format"="%.;%#e HZ;" ("format string")) -> ("error out"=w1306:T13, "String Value Formated"=w1308:T14)  [unwired: 6 in, 1 out]
              n320 = Format Into String(format string="%s; SCOPE LEVSINE; %s, %s", initial string="OUT_IMP " ("format string"), error in=w1306, w1313, w1315, w1308) -> (resulting string=w1311:string, error out=w1312:errorcluster)
              n321 = for {
                N: 2 -> [_]
                tunnel: w1326 -> [w1337]
                tunnel: w1312 -> [w1336]
                tunnel: w1311 -> [w1335]
                tunnel: [w1330] -> w1323
                tunnel: [w1329] -> w1322
                tunnel: w1320 -> [w1334]
                tunnel: w1319 -> [w1333]
                tunnel: w1307 -> [w1328]
                stop <- w1329 continue-if-true
                n322 = call "MLLF_WriteToBuffer.vi"("String"=w1335, "error in"=w1336, "DriverConnect in"=w1337) -> ("error out"=w1332:T13, "DriverConnect out"=w1331:T1)  [unwired: 5 in]
                n323 = call "F5xxx_ESR_check.vi"("Driver Name"=w1333, "Error Code"=w1334, "Model"=w1328, "error in"=w1332, "DriverConnect in"=w1331) -> ("error out"=w1329:T13, "DriverConnect out"=w1330:T1)  [unwired: 5 in]
              }
              n324 = call "Out_On_F5xxx.vi"("DriverConnect in"=w1323, "Model"=w1307, "Output Signal Auto ON"=w1304, "error in"=w1322, "Error Code"=w1320, "Driver Name"=w1319) -> ("error out"=w1321:T13)  [unwired: 8 in, 1 out]
            }
            frame "SCOPE_EDGE", "SCOPEEDGE" {
              # "проверить tdpulse"
              # "ScopeEdge=100k   500m"
              # "SCOPE EDGE; OUT 0.5V, 5 kHz"
              n325 = call "Out_Off_F5xxx.vi"("Driver Name"=w1355, "SwitchOFF"=w1341, "Error Code"=w1356, "Model"=w1343, "DriverConnect in"=w1363) -> ("error out"=w1353:T13, "DriverConnect out"=w1362:T1)  [unwired: 5 in]
              n326 = call "MLLF_FormatStringValue.vi"("error in"=w1353, "String Value"=w1338, "Format"="%.;OUT %#e V" ("format string")) -> ("error out"=w1345:T13, "String Value Formated"=w1351:T14)  [unwired: 6 in, 1 out]
              n327 = call "MLLF_FormatStringValue.vi"("error in"=w1345, "String Value"=w1339, "Format"="%.;%#e HZ;" ("format string")) -> ("error out"=w1342:T13, "String Value Formated"=w1344:T14)  [unwired: 6 in, 1 out]
              n328 = Format Into String(format string="%s; SCOPE EDGE; %s, %s", initial string="OUT_IMP " ("format string"), error in=w1342, w1349, w1351, w1344) -> (resulting string=w1347:string, error out=w1348:errorcluster)
              n329 = for {
                N: 2 -> [_]
                tunnel: w1362 -> [w1373]
                tunnel: w1348 -> [w1372]
                tunnel: w1347 -> [w1371]
                tunnel: [w1366] -> w1359
                tunnel: [w1365] -> w1358
                tunnel: w1356 -> [w1370]
                tunnel: w1355 -> [w1369]
                tunnel: w1343 -> [w1364]
                stop <- w1365 continue-if-true
                n330 = call "MLLF_WriteToBuffer.vi"("String"=w1371, "error in"=w1372, "DriverConnect in"=w1373) -> ("error out"=w1368:T13, "DriverConnect out"=w1367:T1)  [unwired: 5 in]
                n331 = call "F5xxx_ESR_check.vi"("Driver Name"=w1369, "Error Code"=w1370, "Model"=w1364, "error in"=w1368, "DriverConnect in"=w1367) -> ("error out"=w1365:T13, "DriverConnect out"=w1366:T1)  [unwired: 5 in]
              }
              n332 = call "Out_On_F5xxx.vi"("DriverConnect in"=w1359, "Model"=w1343, "Output Signal Auto ON"=w1340, "error in"=w1358, "Error Code"=w1356, "Driver Name"=w1355) -> ("error out"=w1357:T13)  [unwired: 8 in, 1 out]
            }
            frame "SCOPE_MARKER", "SCOPEMARKER" {
              # "проверить работает ли в маркере амплитуда"
              # "ScopeMarker=20n"
              # "SCOPE MARKER; OUT 2 MS"
              n333 = call "Out_Off_F5xxx.vi"("Driver Name"=w1387, "SwitchOFF"=w1375, "Error Code"=w1388, "Model"=w1380, "DriverConnect in"=w1395) -> ("error out"=w1378:T13, "DriverConnect out"=w1394:T1)  [unwired: 5 in]
              n334 = call "MLLF_FormatStringValue.vi"("error in"=w1378, "String Value"=w1377, "Format"="%.; OUT %#e S" ("format string")) -> ("error out"=w1379:T13, "String Value Formated"=w1376:T14)  [unwired: 6 in, 1 out]
              n335 = Format Into String(format string="%s; SCOPE MARKER; %s", initial string="OUT_IMP " ("format string"), error in=w1379, w1384, w1376) -> (resulting string=w1382:string, error out=w1383:errorcluster)
              n336 = for {
                N: 2 -> [_]
                tunnel: w1394 -> [w1405]
                tunnel: w1383 -> [w1404]
                tunnel: w1382 -> [w1403]
                tunnel: [w1398] -> w1391
                tunnel: [w1397] -> w1390
                tunnel: w1388 -> [w1402]
                tunnel: w1387 -> [w1401]
                tunnel: w1380 -> [w1396]
                stop <- w1397 continue-if-true
                n337 = call "MLLF_WriteToBuffer.vi"("String"=w1403, "error in"=w1404, "DriverConnect in"=w1405) -> ("error out"=w1400:T13, "DriverConnect out"=w1399:T1)  [unwired: 5 in]
                n338 = call "F5xxx_ESR_check.vi"("Driver Name"=w1401, "Error Code"=w1402, "Model"=w1396, "error in"=w1400, "DriverConnect in"=w1399) -> ("error out"=w1397:T13, "DriverConnect out"=w1398:T1)  [unwired: 5 in]
              }
              n339 = call "Out_On_F5xxx.vi"("DriverConnect in"=w1391, "Model"=w1380, "Output Signal Auto ON"=w1374, "error in"=w1390, "Error Code"=w1388, "Driver Name"=w1387) -> ("error out"=w1389:T13)  [unwired: 8 in, 1 out]
            }
            frame "<----PQ FUNCTIONS---->" {
            }
            frame "PQ_ CHTONES_NORMAL", "PQ_HURMONICS_NORMAL" {
              w1421 = "H" ("regular expression")
              # "CHTONES PRI"
              # "PQ_ CHTONES_NORMAL=H2 10 0 H3 10 0 H7 30 90 ..."
              n340 = Search and Replace String(replace all?=TRUE ("replace all? (F)"), input string=w1418, search string=w1421, replace string=w1421) -> (number of replacements=w1419:i32)  [unwired: 4 in, 3 out]
              n341 = Match Pattern(string=w1418, regular expression=w1421) -> (after substring=w1420:string)  [unwired: 1 in, 3 out]
              n342 = for {
                N: w1419 -> [_]
                shift-right: [w1430] -> _
                shift-left: w1420 -> [w1429]
                tunnel: [w1428] -> w1422 mode=indexing
                n343 = Match Pattern(string=w1429, regular expression="H") -> (before substring=w1428:string, after substring=w1430:string)  [unwired: 1 in, 2 out]
              }
              n344 = call "MLLF_WriteToBuffer.vi"("String"="PQ OFF;\nPQ CH", "DriverConnect in"=w1410) -> ("error out"=w1407:T13, "DriverConnect out"=w1409:T1)  [unwired: 6 in]
              n345 = for {
                tunnel: [w1444] -> w1417
                tunnel: w1422 -> [w1435] mode=indexing
                tunnel: [w1432] -> w1414
                shift-right: [w1432] -> _
                shift-left: "" -> [w1433]
                tunnel: w1407 -> [_]
                n346 = Match Pattern(string=w1435, regular expression="[\\s\\t]+") -> (before substring=w1449:string, after substring=w1442:string)  [unwired: 1 in, 2 out]
                n347 = Match Pattern(string=w1442, regular expression="[\\s\\t]+") -> (before substring=w1441:string, after substring=w1437:string)  [unwired: 1 in, 2 out]
                n348 = call "MLLF_FormatStringValue.vi"("String Value"=w1449, "Format"=",%.;%#e" ("format")) -> ("error out"=w1448:T13, "String Value Formated"=w1446:T14)  [unwired: 7 in, 1 out]
                n349 = call "MLLF_FormatStringValue.vi"("error in"=w1448, "String Value"=w1441, "Format"=",%.;%#e" ("format")) -> ("error out"=w1439:T13, "String Value Formated"=w1445:T14)  [unwired: 6 in, 1 out]
                n350 = call "MLLF_FormatStringValue.vi"("error in"=w1439, "String Value"=w1437, "Format"=",%.;%#e" ("format")) -> ("error out"=w1438:T13, "String Value Formated"=w1436:T14)  [unwired: 6 in, 1 out]
                n351 = Format Into String(format string="%S%Spct%S", error in=w1438, w1446, w1445, w1436) -> (resulting string=w1434:string, error out=w1444:errorcluster)  [unwired: 1 in]
                n352 = Concatenate Strings(w1433, w1434) -> (w1432:string)
              }
              n353 = Concatenate Strings("CHTONES PRI" ("string"), w1414) -> (w1412:string)
              n354 = for {
                N: 2 -> [_]
                tunnel: w1409 -> [w1462]
                tunnel: w1417 -> [w1461]
                tunnel: [w1455] -> _
                tunnel: [w1456] -> w1424
                tunnel: w1416 -> [w1458]
                tunnel: w1415 -> [w1457]
                tunnel: w1425 -> [w1454]
                tunnel: w1412 -> [w1453]
                stop <- w1456 continue-if-true
                n355 = call "MLLF_WriteToBuffer.vi"("String"=w1453, "error in"=w1461, "DriverConnect in"=w1462) -> ("error out"=w1460:T13, "DriverConnect out"=w1459:T1)  [unwired: 5 in]
                n356 = call "F5xxx_ESR_check.vi"("Driver Name"=w1457, "Error Code"=w1458, "Model"=w1454, "error in"=w1460, "DriverConnect in"=w1459) -> ("error out"=w1456:T13, "DriverConnect out"=w1455:T1)  [unwired: 5 in]
              }
            }
            frame "PQ_ CHTONES_AUX", "PQ_CHTONES_A20", "PQ_HURMONICS_A20", "PQ_HURMONICS_AUX" {
              w1477 = "H" ("regular expression")
              # "CHTONES SEC"
              # "PQ_ CHTONES_AUX=H2 10 0 H3 10 0 H7 30 90 ..."
              n357 = call "MLLF_WriteToBuffer.vi"("String"="\nPQ CH", "DriverConnect in"=w1466) -> ("error out"=w1463:T13, "DriverConnect out"=w1465:T1)  [unwired: 6 in]
              n358 = Match Pattern(string=w1474, regular expression=w1477) -> (after substring=w1476:string)  [unwired: 1 in, 3 out]
              n359 = Search and Replace String(replace all?=TRUE ("replace all? (F)"), input string=w1474, search string=w1477, replace string=w1477) -> (number of replacements=w1475:i32)  [unwired: 4 in, 3 out]
              n360 = for {
                N: w1475 -> [_]
                shift-right: [w1486] -> _
                shift-left: w1476 -> [w1485]
                tunnel: [w1484] -> w1478 mode=indexing
                n361 = Match Pattern(string=w1485, regular expression="H") -> (before substring=w1484:string, after substring=w1486:string)  [unwired: 1 in, 2 out]
              }
              n362 = for {
                tunnel: [w1501] -> w1473
                tunnel: w1478 -> [w1492] mode=indexing
                tunnel: [w1489] -> w1470
                shift-right: [w1489] -> _
                shift-left: "" -> [w1490]
                tunnel: w1463 -> [w1488]
                n363 = Match Pattern(string=w1492, regular expression="[\\s\\t]+") -> (before substring=w1506:string, after substring=w1499:string)  [unwired: 1 in, 2 out]
                n364 = Match Pattern(string=w1499, regular expression="[\\s\\t]+") -> (before substring=w1498:string, after substring=w1494:string)  [unwired: 1 in, 2 out]
                n365 = call "MLLF_FormatStringValue.vi"("error in"=w1488, "String Value"=w1506, "Format"=",%.;%#e" ("format")) -> ("error out"=w1505:T13, "String Value Formated"=w1503:T14)  [unwired: 6 in, 1 out]
                n366 = call "MLLF_FormatStringValue.vi"("error in"=w1505, "String Value"=w1498, "Format"=",%.;%#e" ("format")) -> ("error out"=w1496:T13, "String Value Formated"=w1502:T14)  [unwired: 6 in, 1 out]
                n367 = call "MLLF_FormatStringValue.vi"("error in"=w1496, "String Value"=w1494, "Format"=",%.;%#e" ("format")) -> ("error out"=w1495:T13, "String Value Formated"=w1493:T14)  [unwired: 6 in, 1 out]
                n368 = Format Into String(format string="%S%Spct%S", error in=w1495, w1503, w1502, w1493) -> (resulting string=w1491:string, error out=w1501:errorcluster)  [unwired: 1 in]
                n369 = Concatenate Strings(w1490, w1491) -> (w1489:string)
              }
              n370 = Concatenate Strings("CHTONES PRI" ("string"), w1470) -> (w1468:string)
              n371 = for {
                N: 2 -> [_]
                tunnel: w1465 -> [w1519]
                tunnel: w1473 -> [w1518]
                tunnel: [w1512] -> _
                tunnel: [w1513] -> w1480
                tunnel: w1472 -> [w1515]
                tunnel: w1471 -> [w1514]
                tunnel: w1481 -> [w1511]
                tunnel: w1468 -> [w1510]
                stop <- w1513 continue-if-true
                n372 = call "MLLF_WriteToBuffer.vi"("String"=w1510, "error in"=w1518, "DriverConnect in"=w1519) -> ("error out"=w1517:T13, "DriverConnect out"=w1516:T1)  [unwired: 5 in]
                n373 = call "F5xxx_ESR_check.vi"("Driver Name"=w1514, "Error Code"=w1515, "Model"=w1511, "error in"=w1517, "DriverConnect in"=w1516) -> ("error out"=w1513:T13, "DriverConnect out"=w1512:T1)  [unwired: 5 in]
              }
            }
          }
        }
        frame "get" {
          n374 = Unbundle By Name(w1529) -> ("Permanent data.Connect"=w1523:T1)
          n375 = call "MLLF_CommandDelimeter.vi"("command with param"=w1530) -> ("command"=w1520:string)  [unwired: 6 in, 4 out]
          n376 = case shown="\"VAL\", \"VALUE\"" w1520 {
            selector: w1520 -> [w1532 _ _ _ _ _]
            tunnel: [w1531 _ w1545 w1573 w1589 w1607] -> w1525
            tunnel: w1527 -> [_ _ w1543 w1572 w1588 w1605]
            tunnel: [w1535 w1538 w1560 w1585 w1600 w1622] -> w1528
            tunnel: w1529 -> [w1535 w1538 w1560 w1585 w1600 w1622]
            tunnel: [w1533 w1536 w1541 w1570 w1587 w1603] -> w1524
            tunnel: w1523 -> [_ _ w1553 w1578 w1593 w1615]
            tunnel: w1526 -> [_ _ w1554 w1579 w1594 w1616]
            frame "False", Default {
              n377 = call "MLLF_UnknownCommand(SubVI).vi"("Unknown command"=w1532) -> ("error out"=w1531:errorcluster)  [unwired: 10 in]
              n378 = Build Array(0 ("TimeOut")) -> (w1533:i32[])
            }
            frame "TIMEOUT" {
              n379 = Unbundle By Name(w1538) -> ("Permanent data.Connect.InterfaceSettings.TMO, ms"=w1537:i32)
              n380 = Build Array(w1537) -> (w1536:i32[])
            }
            frame "TC_V", "TC_VOLT", "TCV", "TCVOLT" {
              n381 = call "MLLF_WriteToBuffer.vi"("String"="OUT? V", "DriverConnect in"=w1553) -> ("error out"=w1558:T13, "DriverConnect out"=w1559:T1)  [unwired: 6 in]
              n382 = call "MLLF_ReadBuffer.vi"("Error In"=w1558, "DriverConnect in"=w1559) -> ("Error Out"=w1556:errorcluster, "DriverConnect out"=w1555:T1, "String"=w1542:string)  [unwired: 6 in]
              n383 = Match Pattern(string=w1542, regular expression=",") -> (before substring=w1550:string, after substring=w1548:string)  [unwired: 1 in, 2 out]
              n384 = call "F5xxx_ESR_check.vi"("Driver Name"=w1554, "Error Code"=w1543, "error in"=w1556, "DriverConnect in"=w1555) -> ("error out"=w1544:T13)  [unwired: 6 in, 1 out]
              n385 = Match Pattern(string=w1548, regular expression=",") -> (before substring=w1547:string)  [unwired: 1 in, 3 out]
              n386 = call <vilib>:"Trim Whitespace.vi"("string"=w1547) -> ("trimmed string"=w1546:string)  [unwired: 1 in]
              n387 = case shown="\"False\", Default" w1546 {
                tunnel: w1550 -> [_ w1568]
                tunnel: [_ w1567] -> w1549
                tunnel: w1544 -> [w1565 w1566]
                tunnel: [w1564 w1566] -> w1545
                tunnel: w1543 -> [w1562 _]
                frame "False", Default {
                  n388 = Bundle By Name(cluster=w1565, "source"="Включите режим TC", "code"=w1562, "status"=TRUE) -> (w1564:T13)
                }
                frame "V" {
                  n389 = call <vilib>:"Trim Whitespace.vi"("string"=w1568) -> ("trimmed string"=w1567:string)  [unwired: 1 in]
                }
              }
              n390 = Fract/Exp String To Number(use system decimal point (T)=FALSE, string=w1549) -> (number=w1551:dbl)  [unwired: 2 in, 1 out]
              n391 = Build Array(w1551) -> (w1541:dbl[])
            }
            frame "VAL", "VALUE" {
              n392 = call "MLLF_WriteToBuffer.vi"("String"="OUT?", "DriverConnect in"=w1578) -> ("error out"=w1583:T13, "DriverConnect out"=w1584:T1)  [unwired: 6 in]
              n393 = call "MLLF_ReadBuffer.vi"("Error In"=w1583, "DriverConnect in"=w1584) -> ("Error Out"=w1581:errorcluster, "DriverConnect out"=w1580:T1, "String"=w1571:string)  [unwired: 6 in]
              n394 = call "F5xxx_ESR_check.vi"("Driver Name"=w1579, "Error Code"=w1572, "error in"=w1581, "DriverConnect in"=w1580) -> ("error out"=w1573:T13)  [unwired: 6 in, 1 out]
              n395 = Match Pattern(string=w1571, regular expression=",") -> (before substring=w1575:string)  [unwired: 1 in, 3 out]
              n396 = call <vilib>:"Trim Whitespace.vi"("string"=w1575) -> ("trimmed string"=w1574:string)  [unwired: 1 in]
              n397 = Fract/Exp String To Number(use system decimal point (T)=FALSE, string=w1574) -> (number=w1576:dbl)  [unwired: 2 in, 1 out]
              n398 = Build Array(w1576) -> (w1570:dbl[])
            }
            frame "UNCERTAINTY" {
              n399 = call "MLLF_WriteToBuffer.vi"("String"="UNCERT?", "DriverConnect in"=w1593) -> ("error out"=w1598:T13, "DriverConnect out"=w1599:T1)  [unwired: 6 in]
              n400 = call "MLLF_ReadBuffer.vi"("Error In"=w1598, "DriverConnect in"=w1599) -> ("Error Out"=w1596:errorcluster, "DriverConnect out"=w1595:T1, "String"=w1586:string)  [unwired: 6 in]
              n401 = call "F5xxx_ESR_check.vi"("Driver Name"=w1594, "Error Code"=w1588, "error in"=w1596, "DriverConnect in"=w1595) -> ("error out"=w1589:T13)  [unwired: 6 in, 1 out]
              n402 = call <vilib>:"Trim Whitespace.vi"("string"=w1586) -> ("trimmed string"=w1590:string)  [unwired: 1 in]
              n403 = Fract/Exp String To Number(use system decimal point (T)=FALSE, string=w1590) -> (number=w1591:dbl)  [unwired: 2 in, 1 out]
              n404 = Build Array(w1591) -> (w1587:dbl[])
            }
            frame "RTD_OHM", "RTD_R", "RTDOHM", "RTDR" {
              n405 = call "MLLF_WriteToBuffer.vi"("String"="OUT? OHM", "DriverConnect in"=w1615) -> ("error out"=w1620:T13, "DriverConnect out"=w1621:T1)  [unwired: 6 in]
              n406 = call "MLLF_ReadBuffer.vi"("Error In"=w1620, "DriverConnect in"=w1621) -> ("Error Out"=w1618:errorcluster, "DriverConnect out"=w1617:T1, "String"=w1604:string)  [unwired: 6 in]
              n407 = Match Pattern(string=w1604, regular expression=",") -> (before substring=w1612:string, after substring=w1610:string)  [unwired: 1 in, 2 out]
              n408 = call "F5xxx_ESR_check.vi"("Driver Name"=w1616, "Error Code"=w1605, "error in"=w1618, "DriverConnect in"=w1617) -> ("error out"=w1606:T13)  [unwired: 6 in, 1 out]
              n409 = Match Pattern(string=w1610, regular expression=",") -> (before substring=w1609:string)  [unwired: 1 in, 3 out]
              n410 = call <vilib>:"Trim Whitespace.vi"("string"=w1609) -> ("trimmed string"=w1608:string)  [unwired: 1 in]
              n411 = case shown="\"False\", Default" w1608 {
                tunnel: w1612 -> [_ w1630]
                tunnel: [_ w1629] -> w1611
                tunnel: w1606 -> [w1627 w1628]
                tunnel: [w1626 w1628] -> w1607
                tunnel: w1605 -> [w1624 _]
                frame "False", Default {
                  n412 = Bundle By Name(cluster=w1627, "source"="Включите режим RTD", "code"=w1624, "status"=TRUE) -> (w1626:T13)
                }
                frame "OHM" {
                  n413 = call <vilib>:"Trim Whitespace.vi"("string"=w1630) -> ("trimmed string"=w1629:string)  [unwired: 1 in]
                }
              }
              n414 = Fract/Exp String To Number(use system decimal point (T)=FALSE, string=w1611) -> (number=w1613:dbl)  [unwired: 2 in, 1 out]
              n415 = Build Array(w1613) -> (w1603:dbl[])
            }
          }
          n416 = call "MLLF_FormatOutputValueWithUnits.vi"("error in"=w1525, "ValuesIn"=w1524) -> ("error out"=w1521:T13, "Result string"=w1522:T14)  [unwired: 8 in]
        }
        frame "close" {
          n417 = Unbundle By Name(w1635) -> ("Permanent data.Model"=w1631:dbl)  [unwired: 3 out]
          n418 = call "Out_Off_F5xxx.vi"("Driver Name"=w1633, "Error Code"=w1634, "Model"=w1631) -> ("error out"=w1632:T13)  [unwired: 7 in, 1 out]
          n419 = Unbundle By Name(w1635) -> ("Permanent data.Connect.OpenedSession"=w1637:T3)
          n420 = VISA Close(VISA resource name=w1637, error in (no error)=w1632) -> (error out=w1636:errorcluster)
        }
      }
    }
    frame Error {
    }
  }
  n421 = flat-sequence {
    tunnel: [w1648] -> w6
    tunnel: [w1647] -> w5
    tunnel: w9 -> [w1646]
    tunnel: w7 -> [w1645]
    tunnel: w8 -> [w1641]
    tunnel: [w1643] -> w1
    frame #0 {
      # "driver out"
      n422 = Unbundle By Name(w1641) -> ("Permanent data"=w1640:T17)
      n423 = To Variant(anything=w1640) -> (Variant=w1642:variant)
      n424 = Bundle By Name(cluster=w1641, "Saved Data"=w1642) -> (w1643:T6)
      n425 = call "MLLF_SaveLastSettingUtility.vi"("error in"=w1645, "Saved Data"=w1642) -> ("error out"=w1644:T13)  [unwired: 8 in, 1 out]
      n426 = call "MCF_Output.vi"("Error In"=w1644, "Input"=w1646) -> ("Error Out"=w1647:errorcluster, "Output"=w1648:string)  [unwired: 8 in]
    }
  }
  n427 = local write "Settings"(w1) -> ()
  "error out" <- w5
  "Response" <- w6
